vi "Chip.vi"() -> ()   [LabVIEW 2018]
uses:
  Controls/ClusterF.ctl
  Controls/OpcodeEnum.ctl
  <vilib>/picture/picture.llb/Draw 4-Bit Pixmap.vi
panel:
  out "Display":picture
  # "Keypad                   Keyboard\n+-+-+-+-+                +-+-+-+-+\n|1|2|3|C|                      |1|2|3|4|\n+-+-+-+-+                +-+-+-+-+\n|4|5|6|D|                      |Q|W|E|R|\n+-+-+-+-+     =>     +-+-+-+-+\n|7|8|9|E|                       |A|S|D|F|\n+-+-+-+-+                +-+-+-+-+\n|A|0|B|F|                      |Z|X|C|V|\n+-+-+-+-+                +-+-+-+-+"
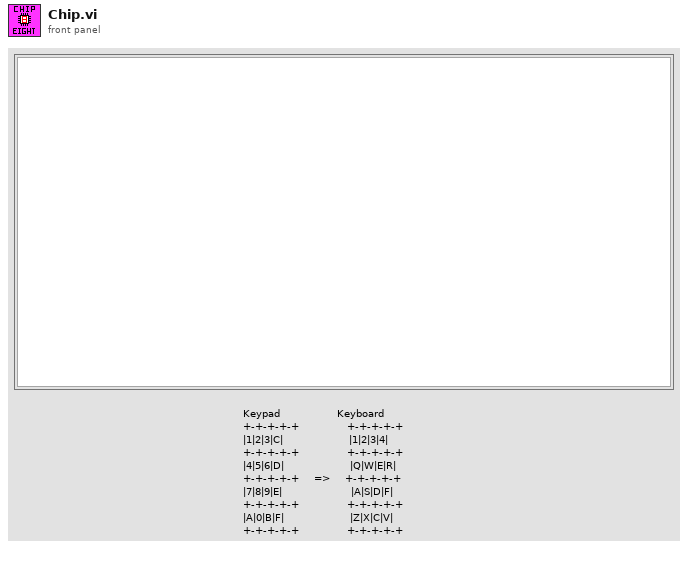
[diagram p1: front panel]
types:
  T1 = typedef "OpcodeEnum.ctl" = enum16{"Initialize", "Load ROM & Fontset", "Fetch Opcode", "Decode Opcode", "Update Display", "Execute Opcode", "Exit Program", "0NNN: Call", "00E0: Clear Display", "00EE: Return from subroutine", "1NNN: Jump to Addr NNN", "2NNN: Call subroutine at NNN", "3XNN: Skip if VX == NN", "4XNN: Skip if VX != NN", "5XY0: Skip if VX = VY", "6XNN: VX = NN", "7XNN: Add NN to VX", "8XY0: VX = VY", "8XY1: VX = VX or VY", "8XY2: VX = VX and VY", "8XY3: VX = VX xor VY", "8XY4: VX += VY", "8XY5: VY - VX", "8XY6: Sig bit of VX to VF, then shift right", "8XY7: Set VX = VY-VX", "8XYE: Sig bit of VX to VF, then shift VX left", "9XY0: Skip if VX != VY", "ANNN: Set I to Addr NNN", "BNNN: Jump to Addr NNN + V0", "CXNN: Set VX to result of rand", "DXYN: Draw Sprite at VX VY (OLD)", "DXYN: Draw Sprite at VX VY", "EX9E: Skip if key stored in VX is pressed", "EXA1: Skip if key stored in VX isn't pressed", "FX07: Set VX to value of DelayTimer", "FX0A: Keypress to VX blocking", "FX15: Set Delay Timer to VX", "FX18: Set SoundTimer to VX", "FX1E: Add VX to I", "FX29: Set Loc of Sprite for VX", "FX33: Store BCD of VX", "FX55: Store V0 to VX", "FX65: Fill V0 to VX", "Debug: Opcode Not Done Yet", "Undefined OpCode"}
  T2 = typedef "ClusterF.ctl" = cluster{"I":u16, "PC":u16, "Memory":u8[], "Keys":u8[], "V Registers":u8[], "Stack":u16[], "StackPointer":u16, "DelayTimer":u8, "SoundTimer":u8, "Display":u8[][], "Opcode":u16, "Display Coords":cluster{"X":u8, "Y":u8}, "GFX":u8[]}
  T3 = enum32{"invalid app kind", "Development System", "Run Time System", "Student Edition", "Embedded LabVIEW", "Evaluation", "Custom"}
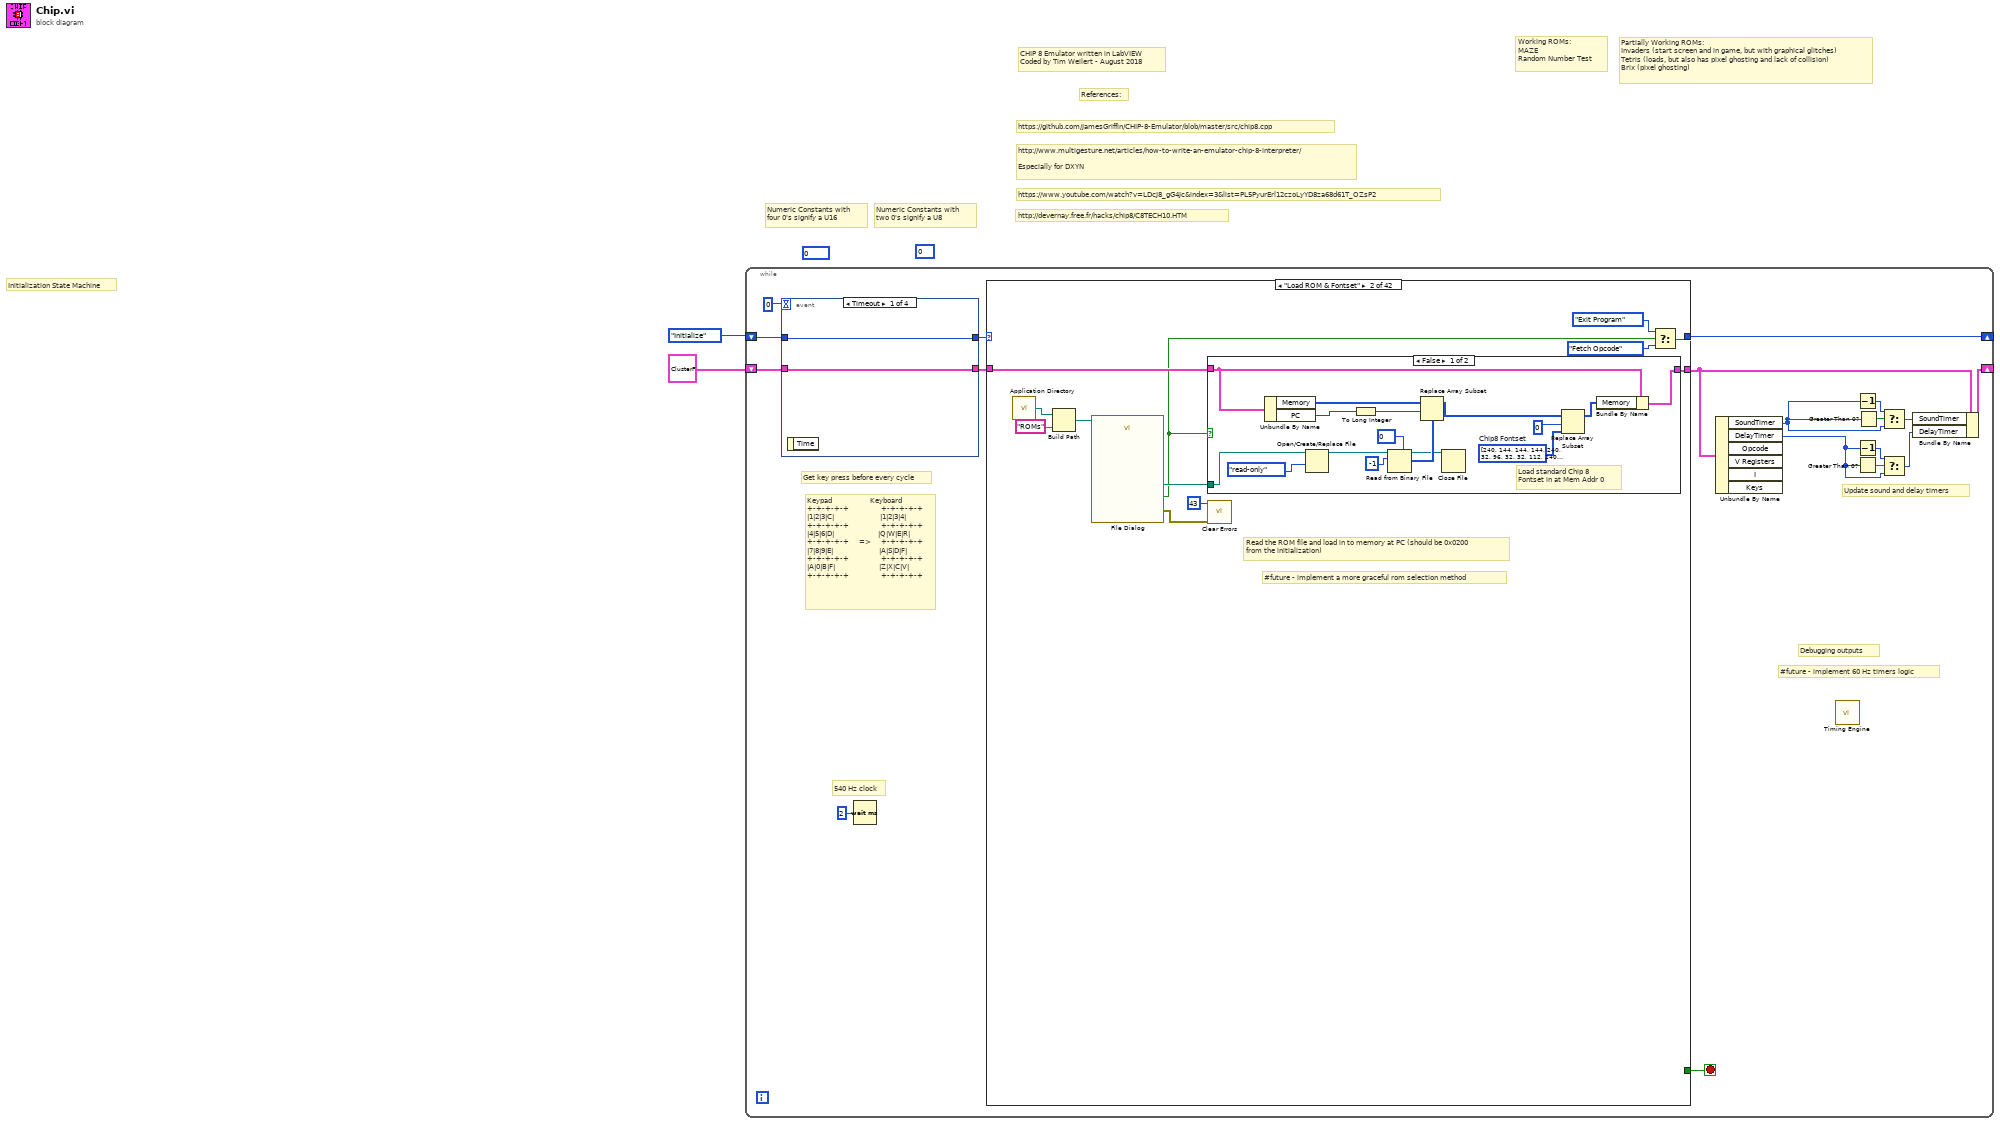
[diagram p0: block diagram]
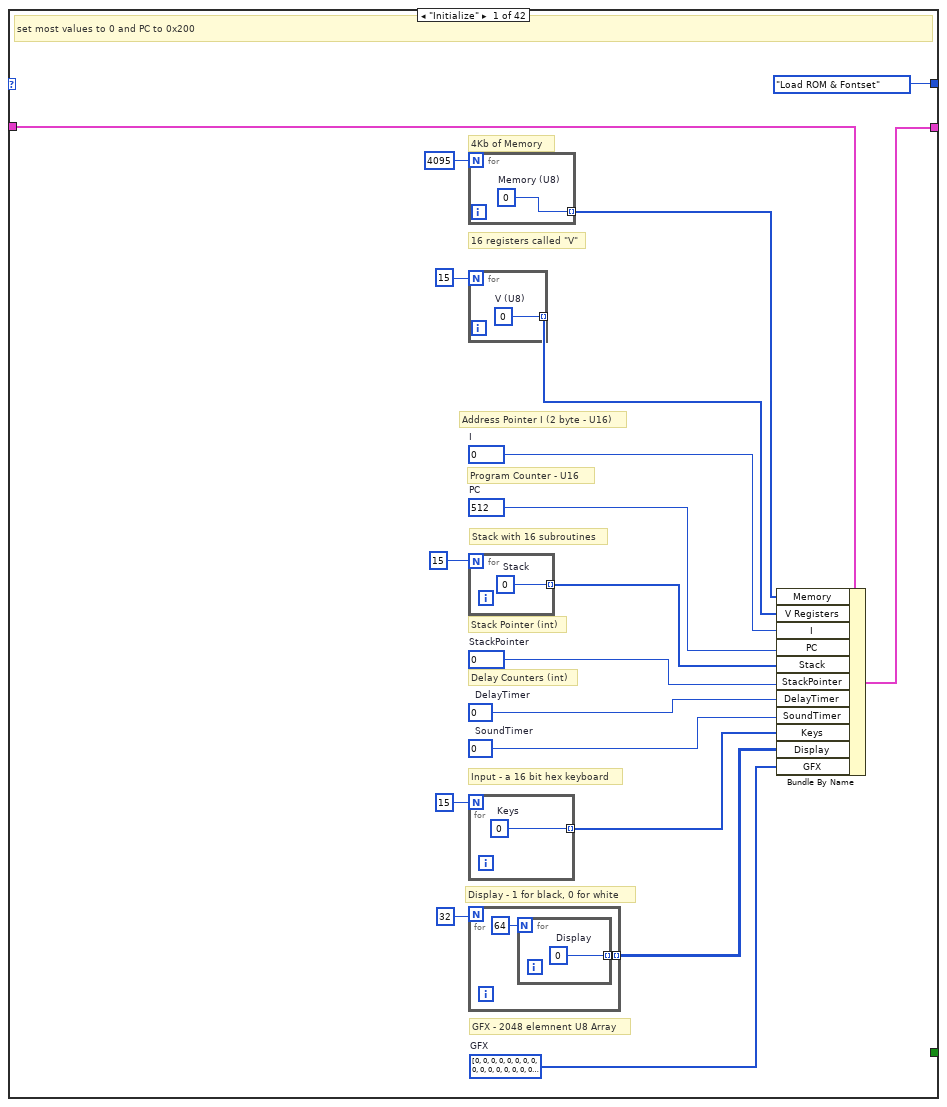
[diagram p2: hidden frame]
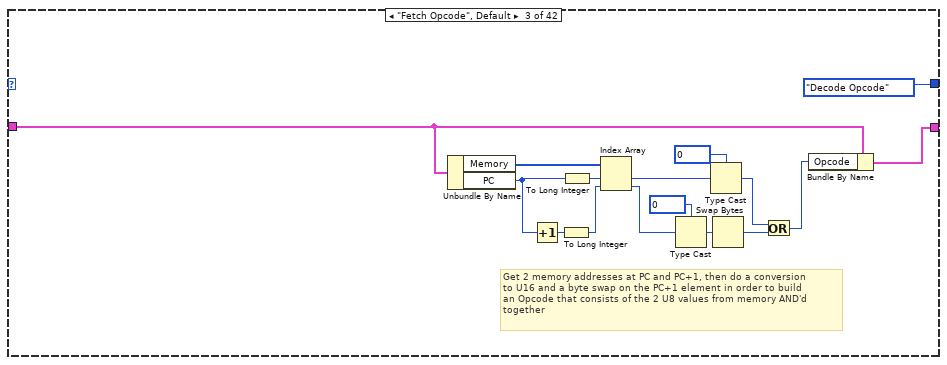
[diagram p4: hidden frame]
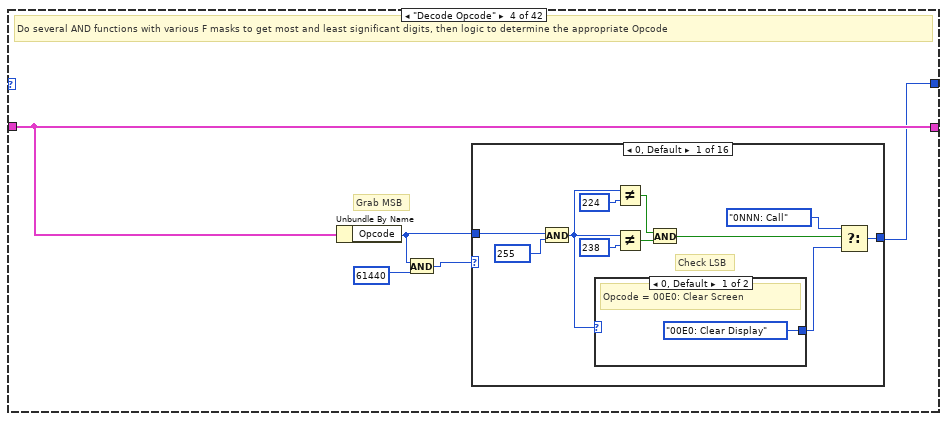
[diagram p5: hidden frame]
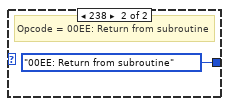
[diagram p6: hidden frame]
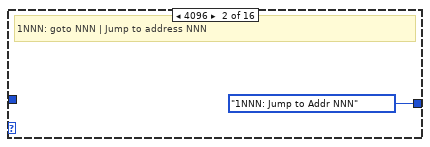
[diagram p7: hidden frame]
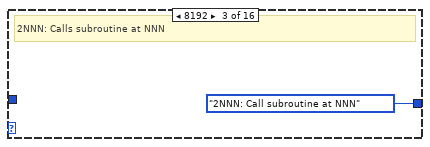
[diagram p8: hidden frame]
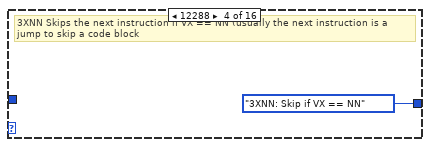
[diagram p9: hidden frame]
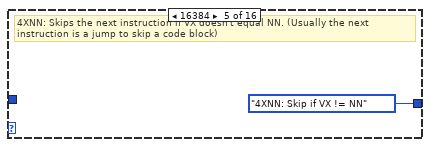
[diagram p10: hidden frame]
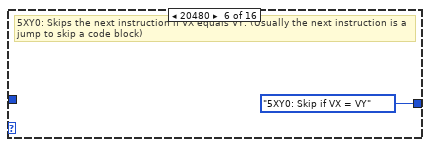
[diagram p11: hidden frame]
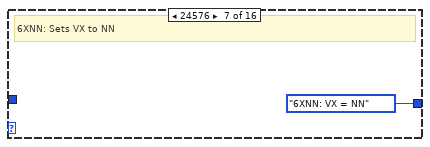
[diagram p12: hidden frame]
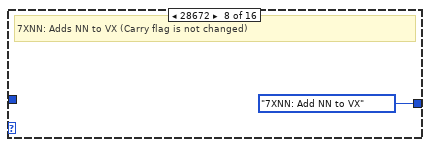
[diagram p13: hidden frame]
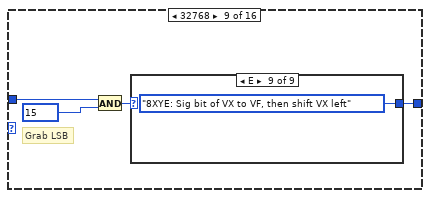
[diagram p14: hidden frame]
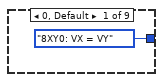
[diagram p15: hidden frame]
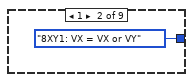
[diagram p16: hidden frame]
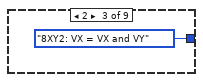
[diagram p17: hidden frame]
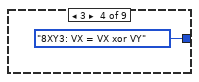
[diagram p18: hidden frame]
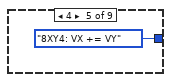
[diagram p19: hidden frame]
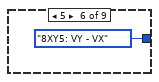
[diagram p20: hidden frame]
diagram:
  (unwired) u8 0
  (unwired) u16 0 ("y")
  # "Partially Working ROMs:\nInvaders (start screen and in game, but with graphical glitches)\nTetris (loads, but also has pixel ghosting and lack of collision)\nBrix (pixel ghosting)"
  # "Working ROMs:\nMAZE\nRandom Number Test"
  # "CHIP 8 Emulator written in LabVIEW\nCoded by Tim Weilert - August 2018"
  # "http://devernay.free.fr/hacks/chip8/C8TECH10.HTM"
  # "References:"
  # "Numeric Constants with \ntwo 0's signify a U8"
  # "Numeric Constants with \nfour 0's signify a U16"
  # "https://github.com/JamesGriffin/CHIP-8-Emulator/blob/master/src/chip8.cpp"
  # "http://www.multigesture.net/articles/how-to-write-an-emulator-chip-8-interpreter/\n\nEspecially for DXYN"
  # "https://www.youtube.com/watch?v=LDcJ8_gG4Jc&index=3&list=PL5PyurErl12czoLyYD8za68d61T_OZsP2"
  # "Initialization State Machine"
  n1 = while {
    shift-right: [w9] -> _
    shift-left: T2 {"I"=0, "PC"=0, "Memory"=array[4095 elements], "Keys"=[0, 0, 0, 0, 0, 0, 0, 0, 0, 0, 0, 0, 0, 0, 0], "V Registers"=[0, 0, 0, 0, 0, 0, 0, 0, 0, 0, 0, 0, 0, 0, 0], "Stack"=[0, 0, 0, 0, 0, 0, 0, 0, 0, 0, 0, 0, 0, 0, 0], "StackPointer"=0, "DelayTimer"=0, "SoundTimer"=0, "Display"=[[0, 0, 0, 0, 0, 0, 0, 0, 0, 0, 0, 0, 0, 0, 0, 0, 0, 0, 0, 0, 0, 0, 0, 0, 0, 0, 0, 0, 0, 0, 0, 0, 0, 0, 0, 0, 0, 0, 0, 0, 0, 0, 0, 0, 0, 0, 0, 0, 0, 0, 0, 0, 0, 0, 0, 0, 0, 0, 0, 0, 0, 0, 0, 0, 0], [0, 0, 0, 0, 0, 0, 0, 0, 0, 0, 0, 0, 0, 0, 0, 0, 0, 0, 0, 0, 0, 0, 0, 0, 0, 0, 0, 0, 0, 0, 0, 0, 0, 0, 0, 0, 0, 0, 0, 0, 0, 0, 0, 0, 0, 0, 0, 0, 0, 0, 0, 0, 0, 0, 0, 0, 0, 0, 0, 0, 0, 0, 0, 0, 0], [0, 0, 0, 0, 0, 0, 0, 0, 0, 0, 0, 0, 0, 0, 0, 0, 0, 0, 0, 0, 0, 0, 0, 0, 0, 0, 0, 0, 0, 0, 0, 0, 0, 0, 0, 0, 0, 0, 0, 0, 0, 0, 0, 0, 0, 0, 0, 0, 0, 0, 0, 0, 0, 0, 0, 0, 0, 0, 0, 0, 0, 0, 0, 0, 0], [0, 0, 0, 0, 0, 0, 0, 0, 0, 0, 0, 0, 0, 0, 0, 0, 0, 0, 0, 0, 0, 0, 0, 0, 0, 0, 0, 0, 0, 0, 0, 0, 0, 0, 0, 0, 0, 0, 0, 0, 0, 0, 0, 0, 0, 0, 0, 0, 0, 0, 0, 0, 0, 0, 0, 0, 0, 0, 0, 0, 0, 0, 0, 0, 0], [0, 0, 0, 0, 0, 0, 0, 0, 0, 0, 0, 0, 0, 0, 0, 0, 0, 0, 0, 0, 0, 0, 0, 0, 0, 0, 0, 0, 0, 0, 0, 0, 0, 0, 0, 0, 0, 0, 0, 0, 0, 0, 0, 0, 0, 0, 0, 0, 0, 0, 0, 0, 0, 0, 0, 0, 0, 0, 0, 0, 0, 0, 0, 0, 0], [0, 0, 0, 0, 0, 0, 0, 0, 0, 0, 0, 0, 0, 0, 0, 0, 0, 0, 0, 0, 0, 0, 0, 0, 0, 0, 0, 0, 0, 0, 0, 0, 0, 0, 0, 0, 0, 0, 0, 0, 0, 0, 0, 0, 0, 0, 0, 0, 0, 0, 0, 0, 0, 0, 0, 0, 0, 0, 0, 0, 0, 0, 0, 0, 0], [0, 0, 0, 0, 0, 0, 0, 0, 0, 0, 0, 0, 0, 0, 0, 0, 0, 0, 0, 0, 0, 0, 0, 0, 0, 0, 0, 0, 0, 0, 0, 0, 0, 0, 0, 0, 0, 0, 0, 0, 0, 0, 0, 0, 0, 0, 0, 0, 0, 0, 0, 0, 0, 0, 0, 0, 0, 0, 0, 0, 0, 0, 0, 0, 0], [0, 0, 0, 0, 0, 0, 0, 0, 0, 0, 0, 0, 0, 0, 0, 0, 0, 0, 0, 0, 0, 0, 0, 0, 0, 0, 0, 0, 0, 0, 0, 0, 0, 0, 0, 0, 0, 0, 0, 0, 0, 0, 0, 0, 0, 0, 0, 0, 0, 0, 0, 0, 0, 0, 0, 0, 0, 0, 0, 0, 0, 0, 0, 0, 0], [0, 0, 0, 0, 0, 0, 0, 0, 0, 0, 0, 0, 0, 0, 0, 0, 0, 0, 0, 0, 0, 0, 0, 0, 0, 0, 0, 0, 0, 0, 0, 0, 0, 0, 0, 0, 0, 0, 0, 0, 0, 0, 0, 0, 0, 0, 0, 0, 0, 0, 0, 0, 0, 0, 0, 0, 0, 0, 0, 0, 0, 0, 0, 0, 0], [0, 0, 0, 0, 0, 0, 0, 0, 0, 0, 0, 0, 0, 0, 0, 0, 0, 0, 0, 0, 0, 0, 0, 0, 0, 0, 0, 0, 0, 0, 0, 0, 0, 0, 0, 0, 0, 0, 0, 0, 0, 0, 0, 0, 0, 0, 0, 0, 0, 0, 0, 0, 0, 0, 0, 0, 0, 0, 0, 0, 0, 0, 0, 0, 0], [0, 0, 0, 0, 0, 0, 0, 0, 0, 0, 0, 0, 0, 0, 0, 0, 0, 0, 0, 0, 0, 0, 0, 0, 0, 0, 0, 0, 0, 0, 0, 0, 0, 0, 0, 0, 0, 0, 0, 0, 0, 0, 0, 0, 0, 0, 0, 0, 0, 0, 0, 0, 0, 0, 0, 0, 0, 0, 0, 0, 0, 0, 0, 0, 0], [0, 0, 0, 0, 0, 0, 0, 0, 0, 0, 0, 0, 0, 0, 0, 0, 0, 0, 0, 0, 0, 0, 0, 0, 0, 0, 0, 0, 0, 0, 0, 0, 0, 0, 0, 0, 0, 0, 0, 0, 0, 0, 0, 0, 0, 0, 0, 0, 0, 0, 0, 0, 0, 0, 0, 0, 0, 0, 0, 0, 0, 0, 0, 0, 0], [0, 0, 0, 0, 0, 0, 0, 0, 0, 0, 0, 0, 0, 0, 0, 0, 0, 0, 0, 0, 0, 0, 0, 0, 0, 0, 0, 0, 0, 0, 0, 0, 0, 0, 0, 0, 0, 0, 0, 0, 0, 0, 0, 0, 0, 0, 0, 0, 0, 0, 0, 0, 0, 0, 0, 0, 0, 0, 0, 0, 0, 0, 0, 0, 0], [0, 0, 0, 0, 0, 0, 0, 0, 0, 0, 0, 0, 0, 0, 0, 0, 0, 0, 0, 0, 0, 0, 0, 0, 0, 0, 0, 0, 0, 0, 0, 0, 0, 0, 0, 0, 0, 0, 0, 0, 0, 0, 0, 0, 0, 0, 0, 0, 0, 0, 0, 0, 0, 0, 0, 0, 0, 0, 0, 0, 0, 0, 0, 0, 0], [0, 0, 0, 0, 0, 0, 0, 0, 0, 0, 0, 0, 0, 0, 0, 0, 0, 0, 0, 0, 0, 0, 0, 0, 0, 0, 0, 0, 0, 0, 0, 0, 0, 0, 0, 0, 0, 0, 0, 0, 0, 0, 0, 0, 0, 0, 0, 0, 0, 0, 0, 0, 0, 0, 0, 0, 0, 0, 0, 0, 0, 0, 0, 0, 0], [0, 0, 0, 0, 0, 0, 0, 0, 0, 0, 0, 0, 0, 0, 0, 0, 0, 0, 0, 0, 0, 0, 0, 0, 0, 0, 0, 0, 0, 0, 0, 0, 0, 0, 0, 0, 0, 0, 0, 0, 0, 0, 0, 0, 0, 0, 0, 0, 0, 0, 0, 0, 0, 0, 0, 0, 0, 0, 0, 0, 0, 0, 0, 0, 0], [0, 0, 0, 0, 0, 0, 0, 0, 0, 0, 0, 0, 0, 0, 0, 0, 0, 0, 0, 0, 0, 0, 0, 0, 0, 0, 0, 0, 0, 0, 0, 0, 0, 0, 0, 0, 0, 0, 0, 0, 0, 0, 0, 0, 0, 0, 0, 0, 0, 0, 0, 0, 0, 0, 0, 0, 0, 0, 0, 0, 0, 0, 0, 0, 0], [0, 0, 0, 0, 0, 0, 0, 0, 0, 0, 0, 0, 0, 0, 0, 0, 0, 0, 0, 0, 0, 0, 0, 0, 0, 0, 0, 0, 0, 0, 0, 0, 0, 0, 0, 0, 0, 0, 0, 0, 0, 0, 0, 0, 0, 0, 0, 0, 0, 0, 0, 0, 0, 0, 0, 0, 0, 0, 0, 0, 0, 0, 0, 0, 0], [0, 0, 0, 0, 0, 0, 0, 0, 0, 0, 0, 0, 0, 0, 0, 0, 0, 0, 0, 0, 0, 0, 0, 0, 0, 0, 0, 0, 0, 0, 0, 0, 0, 0, 0, 0, 0, 0, 0, 0, 0, 0, 0, 0, 0, 0, 0, 0, 0, 0, 0, 0, 0, 0, 0, 0, 0, 0, 0, 0, 0, 0, 0, 0, 0], [0, 0, 0, 0, 0, 0, 0, 0, 0, 0, 0, 0, 0, 0, 0, 0, 0, 0, 0, 0, 0, 0, 0, 0, 0, 0, 0, 0, 0, 0, 0, 0, 0, 0, 0, 0, 0, 0, 0, 0, 0, 0, 0, 0, 0, 0, 0, 0, 0, 0, 0, 0, 0, 0, 0, 0, 0, 0, 0, 0, 0, 0, 0, 0, 0], [0, 0, 0, 0, 0, 0, 0, 0, 0, 0, 0, 0, 0, 0, 0, 0, 0, 0, 0, 0, 0, 0, 0, 0, 0, 0, 0, 0, 0, 0, 0, 0, 0, 0, 0, 0, 0, 0, 0, 0, 0, 0, 0, 0, 0, 0, 0, 0, 0, 0, 0, 0, 0, 0, 0, 0, 0, 0, 0, 0, 0, 0, 0, 0, 0], [0, 0, 0, 0, 0, 0, 0, 0, 0, 0, 0, 0, 0, 0, 0, 0, 0, 0, 0, 0, 0, 0, 0, 0, 0, 0, 0, 0, 0, 0, 0, 0, 0, 0, 0, 0, 0, 0, 0, 0, 0, 0, 0, 0, 0, 0, 0, 0, 0, 0, 0, 0, 0, 0, 0, 0, 0, 0, 0, 0, 0, 0, 0, 0, 0], [0, 0, 0, 0, 0, 0, 0, 0, 0, 0, 0, 0, 0, 0, 0, 0, 0, 0, 0, 0, 0, 0, 0, 0, 0, 0, 0, 0, 0, 0, 0, 0, 0, 0, 0, 0, 0, 0, 0, 0, 0, 0, 0, 0, 0, 0, 0, 0, 0, 0, 0, 0, 0, 0, 0, 0, 0, 0, 0, 0, 0, 0, 0, 0, 0], [0, 0, 0, 0, 0, 0, 0, 0, 0, 0, 0, 0, 0, 0, 0, 0, 0, 0, 0, 0, 0, 0, 0, 0, 0, 0, 0, 0, 0, 0, 0, 0, 0, 0, 0, 0, 0, 0, 0, 0, 0, 0, 0, 0, 0, 0, 0, 0, 0, 0, 0, 0, 0, 0, 0, 0, 0, 0, 0, 0, 0, 0, 0, 0, 0], [0, 0, 0, 0, 0, 0, 0, 0, 0, 0, 0, 0, 0, 0, 0, 0, 0, 0, 0, 0, 0, 0, 0, 0, 0, 0, 0, 0, 0, 0, 0, 0, 0, 0, 0, 0, 0, 0, 0, 0, 0, 0, 0, 0, 0, 0, 0, 0, 0, 0, 0, 0, 0, 0, 0, 0, 0, 0, 0, 0, 0, 0, 0, 0, 0], [0, 0, 0, 0, 0, 0, 0, 0, 0, 0, 0, 0, 0, 0, 0, 0, 0, 0, 0, 0, 0, 0, 0, 0, 0, 0, 0, 0, 0, 0, 0, 0, 0, 0, 0, 0, 0, 0, 0, 0, 0, 0, 0, 0, 0, 0, 0, 0, 0, 0, 0, 0, 0, 0, 0, 0, 0, 0, 0, 0, 0, 0, 0, 0, 0], [0, 0, 0, 0, 0, 0, 0, 0, 0, 0, 0, 0, 0, 0, 0, 0, 0, 0, 0, 0, 0, 0, 0, 0, 0, 0, 0, 0, 0, 0, 0, 0, 0, 0, 0, 0, 0, 0, 0, 0, 0, 0, 0, 0, 0, 0, 0, 0, 0, 0, 0, 0, 0, 0, 0, 0, 0, 0, 0, 0, 0, 0, 0, 0, 0], [0, 0, 0, 0, 0, 0, 0, 0, 0, 0, 0, 0, 0, 0, 0, 0, 0, 0, 0, 0, 0, 0, 0, 0, 0, 0, 0, 0, 0, 0, 0, 0, 0, 0, 0, 0, 0, 0, 0, 0, 0, 0, 0, 0, 0, 0, 0, 0, 0, 0, 0, 0, 0, 0, 0, 0, 0, 0, 0, 0, 0, 0, 0, 0, 0], [0, 0, 0, 0, 0, 0, 0, 0, 0, 0, 0, 0, 0, 0, 0, 0, 0, 0, 0, 0, 0, 0, 0, 0, 0, 0, 0, 0, 0, 0, 0, 0, 0, 0, 0, 0, 0, 0, 0, 0, 0, 0, 0, 0, 0, 0, 0, 0, 0, 0, 0, 0, 0, 0, 0, 0, 0, 0, 0, 0, 0, 0, 0, 0, 0], [0, 0, 0, 0, 0, 0, 0, 0, 0, 0, 0, 0, 0, 0, 0, 0, 0, 0, 0, 0, 0, 0, 0, 0, 0, 0, 0, 0, 0, 0, 0, 0, 0, 0, 0, 0, 0, 0, 0, 0, 0, 0, 0, 0, 0, 0, 0, 0, 0, 0, 0, 0, 0, 0, 0, 0, 0, 0, 0, 0, 0, 0, 0, 0, 0], [0, 0, 0, 0, 0, 0, 0, 0, 0, 0, 0, 0, 0, 0, 0, 0, 0, 0, 0, 0, 0, 0, 0, 0, 0, 0, 0, 0, 0, 0, 0, 0, 0, 0, 0, 0, 0, 0, 0, 0, 0, 0, 0, 0, 0, 0, 0, 0, 0, 0, 0, 0, 0, 0, 0, 0, 0, 0, 0, 0, 0, 0, 0, 0, 0], [0, 0, 0, 0, 0, 0, 0, 0, 0, 0, 0, 0, 0, 0, 0, 0, 0, 0, 0, 0, 0, 0, 0, 0, 0, 0, 0, 0, 0, 0, 0, 0, 0, 0, 0, 0, 0, 0, 0, 0, 0, 0, 0, 0, 0, 0, 0, 0, 0, 0, 0, 0, 0, 0, 0, 0, 0, 0, 0, 0, 0, 0, 0, 0, 0], [0, 0, 0, 0, 0, 0, 0, 0, 0, 0, 0, 0, 0, 0, 0, 0, 0, 0, 0, 0, 0, 0, 0, 0, 0, 0, 0, 0, 0, 0, 0, 0, 0, 0, 0, 0, 0, 0, 0, 0, 0, 0, 0, 0, 0, 0, 0, 0, 0, 0, 0, 0, 0, 0, 0, 0, 0, 0, 0, 0, 0, 0, 0, 0, 0]], "Opcode"=0, "Display Coords"={"X"=0, "Y"=0}, "GFX"=[]} ("Variables and Memory") -> [w18]
    shift-right: [w5] -> _
    shift-left: OpcodeEnum."Initialize" -> [w4]
    stop <- w20 stop-if-true
    # "#future - implement 60 Hz timers logic"
    # "Debugging outputs"
    # "Update sound and delay timers"
    # "540 Hz clock"
    # "Get key press before every cycle"
    # "Keypad                   Keyboard\n+-+-+-+-+                +-+-+-+-+\n|1|2|3|C|                       |1|2|3|4|\n+-+-+-+-+                +-+-+-+-+\n|4|5|6|D|                      |Q|W|E|R|\n+-+-+-+-+     =>     +-+-+-+-+\n|7|8|9|E|                       |A|S|D|F|\n+-+-+-+-+                +-+-+-+-+\n|A|0|B|F|                      |Z|X|C|V|\n+-+-+-+-+                +-+-+-+-+"
    n2 = event shown="[0] Timeout" {
      selector: _ -> [_ _ _ _]
      dyn-events: _ -> [_ _ _ _]
      timeout: 0 -> [_ _ _ _]
      tunnel: w18 -> [w788 w789 w795 w799]
      tunnel: [w788 w789 w793 w800] -> w17
      tunnel: w4 -> [w787 _ w792 w796]
      tunnel: [w787 OpcodeEnum."Exit Program" w792 w796] -> w3
      event Timeout {
        n3 = event-data() -> ()  [unwired: 1 in, 1 out]
      }
      event Panel Close? {
        n4 = event-data() -> ()  [unwired: 1 in, 1 out]
        n5 = event-data("Discard?"=TRUE) -> ()  [unwired: 1 in, 1 out]
      }
      event Key Up {
        n6 = event-data() -> ()  [unwired: 1 in, 1 out]
        n7 = Bundle By Name(cluster=w795, "Keys"=u8[] [0, 0, 0, 0, 0, 0, 0, 0, 0, 0, 0, 0, 0, 0, 0, 0]) -> (w793:T2)
      }
      event Key Down {
        n8 = event-data() -> ("Char"=w798:i16)  [unwired: 1 in]
        n9 = case shown="78" w798 {
          tunnel: [u8[] [0, 0, 0, 0, 0, 0, 0, 0, 0, 0, 0, 0, 0, 0, 0, 0] ("Keys 2") u8[] [0, 1, 0, 0, 0, 0, 0, 0, 0, 0, 0, 0, 0, 0, 0, 0] ("Keys 2") u8[] [0, 0, 1, 0, 0, 0, 0, 0, 0, 0, 0, 0, 0, 0, 0, 0] ("Keys 2") u8[] [0, 0, 0, 1, 0, 0, 0, 0, 0, 0, 0, 0, 0, 0, 0, 0] ("Keys 2") u8[] [0, 0, 0, 0, 0, 0, 0, 0, 0, 0, 0, 0, 1, 0, 0, 0] ("Keys 2") u8[] [0, 0, 0, 0, 1, 0, 0, 0, 0, 0, 0, 0, 0, 0, 0, 0] ("Keys 2") u8[] [0, 0, 0, 0, 0, 1, 0, 0, 0, 0, 0, 0, 0, 0, 0, 0] ("Keys 2") u8[] [0, 0, 0, 0, 0, 0, 1, 0, 0, 0, 0, 0, 0, 0, 0, 0] ("Keys 2") u8[] [0, 0, 0, 0, 0, 0, 0, 0, 0, 0, 0, 0, 0, 1, 0, 0] ("Keys 2") u8[] [0, 0, 0, 0, 0, 0, 0, 1, 0, 0, 0, 0, 0, 0, 0, 0] ("Keys 2") u8[] [0, 0, 0, 0, 0, 0, 0, 0, 1, 0, 0, 0, 0, 0, 0, 0] ("Keys 2") u8[] [0, 0, 0, 0, 0, 0, 0, 0, 0, 1, 0, 0, 0, 0, 0, 0] ("Keys 2") u8[] [0, 0, 0, 0, 0, 0, 0, 0, 0, 0, 0, 0, 0, 0, 1, 0] ("Keys 2") u8[] [0, 0, 0, 0, 0, 0, 0, 0, 0, 0, 1, 0, 0, 0, 0, 0] ("Keys 2") u8[] [1, 0, 0, 0, 0, 0, 0, 0, 0, 0, 0, 0, 0, 0, 0, 0] ("Keys 2") u8[] [0, 0, 0, 0, 0, 0, 0, 0, 0, 0, 0, 1, 0, 0, 0, 0] ("Keys 2") u8[] [0, 0, 0, 0, 0, 0, 0, 0, 0, 0, 0, 0, 0, 0, 0, 1] ("Keys 2")] -> w797
          frame 0, Default {
          }
          frame 49 {
            # "1 = 1"
          }
          frame 50 {
            # "2 = 2"
          }
          frame 51 {
            # "3 = 3"
          }
          frame 52 {
            # "4 =C"
          }
          frame 113 {
            # "Q = 4"
          }
          frame 119 {
            # "W = 5"
          }
          frame 101 {
            # "E = 6"
          }
          frame 114 {
            # "R = D"
          }
          frame 97 {
            # "A = 7"
          }
          frame 115 {
            # "S = 8"
          }
          frame 100 {
            # "D = 9"
          }
          frame 102 {
            # "F = E"
          }
          frame 122 {
            # "Z = A"
          }
          frame 120 {
            # "X = 0"
          }
          frame 99 {
            # "C = B"
          }
          frame 118 {
            # "V = F"
          }
        }
        n10 = Bundle By Name(cluster=w799, "Keys"=w797) -> (w800:T2)
      }
    }
    n11 = Wait (ms)(milliseconds to wait=u32 2) -> ()  [unwired: 1 out]
    n12 = case shown="\"Load ROM & Fontset\"" w3 {
      tunnel: w17 -> [w22 w58 w89 w96 w159 w162 w167 w177 w189 w198 w205 w226 w235 w259 w275 w285 w308 w328 w338 w354 w384 w402 w423 w453 w474 w495 w507 w511 w530 w546 w557 w585 w599 w602 w652 w657 w685 w702 w735 w754 w771 w783]
      tunnel: [w23 w57 w88 w96 w159 w162 w168 w178 w190 w197 w206 w227 w233 w258 w276 w286 w309 w327 w337 w355 w385 w401 w422 w454 w473 w494 w508 w512 w531 w548 w558 w584 w600 w608 w653 w658 w686 w703 w736 w755 w770 w783] -> w10
      tunnel: [OpcodeEnum."Load ROM & Fontset" w50 OpcodeEnum."Decode Opcode" w93 OpcodeEnum."Fetch Opcode" OpcodeEnum."Exit Program" OpcodeEnum."Fetch Opcode" OpcodeEnum."Update Display" OpcodeEnum."Fetch Opcode" OpcodeEnum."Fetch Opcode" OpcodeEnum."Fetch Opcode" OpcodeEnum."Fetch Opcode" OpcodeEnum."Fetch Opcode" OpcodeEnum."Fetch Opcode" OpcodeEnum."Fetch Opcode" OpcodeEnum."Fetch Opcode" OpcodeEnum."Fetch Opcode" OpcodeEnum."Fetch Opcode" OpcodeEnum."Fetch Opcode" OpcodeEnum."Fetch Opcode" OpcodeEnum."Fetch Opcode" OpcodeEnum."Fetch Opcode" OpcodeEnum."Fetch Opcode" OpcodeEnum."Fetch Opcode" OpcodeEnum."Fetch Opcode" OpcodeEnum."Fetch Opcode" OpcodeEnum."Fetch Opcode" OpcodeEnum."Fetch Opcode" OpcodeEnum."Fetch Opcode" OpcodeEnum."Update Display" OpcodeEnum."Fetch Opcode" OpcodeEnum."Fetch Opcode" OpcodeEnum."Fetch Opcode" OpcodeEnum."Fetch Opcode" OpcodeEnum."Fetch Opcode" OpcodeEnum."Fetch Opcode" OpcodeEnum."Fetch Opcode" OpcodeEnum."Fetch Opcode" OpcodeEnum."Fetch Opcode" OpcodeEnum."Fetch Opcode" OpcodeEnum."Fetch Opcode" OpcodeEnum."Debug: Opcode Not Done Yet"] -> w5
      tunnel: [_ _ _ _ _ TRUE _ _ _ _ _ _ _ _ _ _ _ _ _ _ _ _ _ _ _ _ _ _ _ FALSE _ _ _ _ _ _ _ _ _ _ _ TRUE] -> w20
      frame "Initialize" {
        w24 = u8[] [0, 0, 0, 0, 0, 0, 0, 0, 0, 0, 0, 0, 0, 0, 0, 0, 0, 0, 0, 0, 0, 0, 0, 0, 0, 0, 0, 0, 0, 0, 0, 0, 0, 0, 0, 0, 0, 0, 0, 0, 0, 0, 0, 0, 0, 0, 0, 0, 0, 0, 0, 0, 0, 0, 0, 0, 0, 0, 0, 0, 0, 0, 0, 0, 0, 0, 0, 0, 0, 0, 0, 0, 0, 0, 0, 0, 0, 0, 0, 0, 0, 0, 0, 0, 0, 0, 0, 0, 0, 0, 0, 0, 0, 0, 0, 0, 0, 0, 0, 0, 0, 0, 0, 0, 0, 0, 0, 0, 0, 0, 0, 0, 0, 0, 0, 0, 0, 0, 0, 0, 0, 0, 0, 0, 0, 0, 0, 0, 0, 0, 0, 0, 0, 0, 0, 0, 0, 0, 0, 0, 0, 0, 0, 0, 0, 0, 0, 0, 0, 0, 0, 0, 0, 0, 0, 0, 0, 0, 0, 0, 0, 0, 0, 0, 0, 0, 0, 0, 0, 0, 0, 0, 0, 0, 0, 0, 0, 0, 0, 0, 0, 0, 0, 0, 0, 0, 0, 0, 0, 0, 0, 0, 0, 0, 0, 0, 0, 0, 0, 0, 0, 0, 0, 0, 0, 0, 0, 0, 0, 0, 0, 0, 0, 0, 0, 0, 0, 0, 0, 0, 0, 0, 0, 0, 0, 0, 0, 0, 0, 0, 0, 0, 0, 0, 0, 0, 0, 0, 0, 0, 0, 0, 0, 0, 0, 0, 0, 0, 0, 0, 0, 0, 0, 0, 0, 0, 0, 0, 0, 0, 0, 0, 0, 0, 0, 0, 0, 0, 0, 0, 0, 0, 0, 0, 0, 0, 0, 0, 0, 0, 0, 0, 0, 0, 0, 0, 0, 0, 0, 0, 0, 0, 0, 0, 0, 0, 0, 0, 0, 0, 0, 0, 0, 0, 0, 0, 0, 0, 0, 0, 0, 0, 0, 0, 0, 0, 0, 0, 0, 0, 0, 0, 0, 0, 0, 0, 0, 0, 0, 0, 0, 0, 0, 0, 0, 0, 0, 0, 0, 0, 0, 0, 0, 0, 0, 0, 0, 0, 0, 0, 0, 0, 0, 0, 0, 0, 0, 0, 0, 0, 0, 0, 0, 0, 0, 0, 0, 0, 0, 0, 0, 0, 0, 0, 0, 0, 0, 0, 0, 0, 0, 0, 0, 0, 0, 0, 0, 0, 0, 0, 0, 0, 0, 0, 0, 0, 0, 0, 0, 0, 0, 0, 0, 0, 0, 0, 0, 0, 0, 0, 0, 0, 0, 0, 0, 0, 0, 0, 0, 0, 0, 0, 0, 0, 0, 0, 0, 0, 0, 0, 0, 0, 0, 0, 0, 0, 0, 0, 0, 0, 0, 0, 0, 0, 0, 0, 0, 0, 0, 0, 0, 0, 0, 0, 0, 0, 0, 0, 0, 0, 0, 0, 0, 0, 0, 0, 0, 0, 0, 0, 0, 0, 0, 0, 0, 0, 0, 0, 0, 0, 0, 0, 0, 0, 0, 0, 0, 0, 0, 0, 0, 0, 0, 0, 0, 0, 0, 0, 0, 0, 0, 0, 0, 0, 0, 0, 0, 0, 0, 0, 0, 0, 0, 0, 0, 0, 0, 0, 0, 0, 0, 0, 0, 0, 0, 0, 0, 0, 0, 0, 0, 0, 0, 0, 0, 0, 0, 0, 0, 0, 0, 0, 0, 0, 0, 0, 0, 0, 0, 0, 0, 0, 0, 0, 0, 0, 0, 0, 0, 0, 0, 0, 0, 0, 0, 0, 0, 0, 0, 0, 0, 0, 0, 0, 0, 0, 0, 0, 0, 0, 0, 0, 0, 0, 0, 0, 0, 0, 0, 0, 0, 0, 0, 0, 0, 0, 0, 0, 0, 0, 0, 0, 0, 0, 0, 0, 0, 0, 0, 0, 0, 0, 0, 0, 0, 0, 0, 0, 0, 0, 0, 0, 0, 0, 0, 0, 0, 0, 0, 0, 0, 0, 0, 0, 0, 0, 0, 0, 0, 0, 0, 0, 0, 0, 0, 0, 0, 0, 0, 0, 0, 0, 0, 0, 0, 0, 0, 0, 0, 0, 0, 0, 0, 0, 0, 0, 0, 0, 0, 0, 0, 0, 0, 0, 0, 0, 0, 0, 0, 0, 0, 0, 0, 0, 0, 0, 0, 0, 0, 0, 0, 0, 0, 0, 0, 0, 0, 0, 0, 0, 0, 0, 0, 0, 0, 0, 0, 0, 0, 0, 0, 0, 0, 0, 0, 0, 0, 0, 0, 0, 0, 0, 0, 0, 0, 0, 0, 0, 0, 0, 0, 0, 0, 0, 0, 0, 0, 0, 0, 0, 0, 0, 0, 0, 0, 0, 0, 0, 0, 0, 0, 0, 0, 0, 0, 0, 0, 0, 0, 0, 0, 0, 0, 0, 0, 0, 0, 0, 0, 0, 0, 0, 0, 0, 0, 0, 0, 0, 0, 0, 0, 0, 0, 0, 0, 0, 0, 0, 0, 0, 0, 0, 0, 0, 0, 0, 0, 0, 0, 0, 0, 0, 0, 0, 0, 0, 0, 0, 0, 0, 0, 0, 0, 0, 0, 0, 0, 0, 0, 0, 0, 0, 0, 0, 0, 0, 0, 0, 0, 0, 0, 0, 0, 0, 0, 0, 0, 0, 0, 0, 0, 0, 0, 0, 0, 0, 0, 0, 0, 0, 0, 0, 0, 0, 0, 0, 0, 0, 0, 0, 0, 0, 0, 0, 0, 0, 0, 0, 0, 0, 0, 0, 0, 0, 0, 0, 0, 0, 0, 0, 0, 0, 0, 0, 0, 0, 0, 0, 0, 0, 0, 0, 0, 0, 0, 0, 0, 0, 0, 0, 0, 0, 0, 0, 0, 0, 0, 0, 0, 0, 0, 0, 0, 0, 0, 0, 0, 0, 0, 0, 0, 0, 0, 0, 0, 0, 0, 0, 0, 0, 0, 0, 0, 0, 0, 0, 0, 0, 0, 0, 0, 0, 0, 0, 0, 0, 0, 0, 0, 0, 0, 0, 0, 0, 0, 0, 0, 0, 0, 0, 0, 0, 0, 0, 0, 0, 0, 0, 0, 0, 0, 0, 0, 0, 0, 0, 0, 0, 0, 0, 0, 0, 0, 0, 0, 0, 0, 0, 0, 0, 0, 0, 0, 0, 0, 0, 0, 0, 0, 0, 0, 0, 0, 0, 0, 0, 0, 0, 0, 0, 0, 0, 0, 0, 0, 0, 0, 0, 0, 0, 0, 0, 0, 0, 0, 0, 0, 0, 0, 0, 0, 0, 0, 0, 0, 0, 0, 0, 0, 0, 0, 0, 0, 0, 0, 0, 0, 0, 0, 0, 0, 0, 0, 0, 0, 0, 0, 0, 0, 0, 0, 0, 0, 0, 0, 0, 0, 0, 0, 0, 0, 0, 0, 0, 0, 0, 0, 0, 0, 0, 0, 0, 0, 0, 0, 0, 0, 0, 0, 0, 0, 0, 0, 0, 0, 0, 0, 0, 0, 0, 0, 0, 0, 0, 0, 0, 0, 0, 0, 0, 0, 0, 0, 0, 0, 0, 0, 0, 0, 0, 0, 0, 0, 0, 0, 0, 0, 0, 0, 0, 0, 0, 0, 0, 0, 0, 0, 0, 0, 0, 0, 0, 0, 0, 0, 0, 0, 0, 0, 0, 0, 0, 0, 0, 0, 0, 0, 0, 0, 0, 0, 0, 0, 0, 0, 0, 0, 0, 0, 0, 0, 0, 0, 0, 0, 0, 0, 0, 0, 0, 0, 0, 0, 0, 0, 0, 0, 0, 0, 0, 0, 0, 0, 0, 0, 0, 0, 0, 0, 0, 0, 0, 0, 0, 0, 0, 0, 0, 0, 0, 0, 0, 0, 0, 0, 0, 0, 0, 0, 0, 0, 0, 0, 0, 0, 0, 0, 0, 0, 0, 0, 0, 0, 0, 0, 0, 0, 0, 0, 0, 0, 0, 0, 0, 0, 0, 0, 0, 0, 0, 0, 0, 0, 0, 0, 0, 0, 0, 0, 0, 0, 0, 0, 0, 0, 0, 0, 0, 0, 0, 0, 0, 0, 0, 0, 0, 0, 0, 0, 0, 0, 0, 0, 0, 0, 0, 0, 0, 0, 0, 0, 0, 0, 0, 0, 0, 0, 0, 0, 0, 0, 0, 0, 0, 0, 0, 0, 0, 0, 0, 0, 0, 0, 0, 0, 0, 0, 0, 0, 0, 0, 0, 0, 0, 0, 0, 0, 0, 0, 0, 0, 0, 0, 0, 0, 0, 0, 0, 0, 0, 0, 0, 0, 0, 0, 0, 0, 0, 0, 0, 0, 0, 0, 0, 0, 0, 0, 0, 0, 0, 0, 0, 0, 0, 0, 0, 0, 0, 0, 0, 0, 0, 0, 0, 0, 0, 0, 0, 0, 0, 0, 0, 0, 0, 0, 0, 0, 0, 0, 0, 0, 0, 0, 0, 0, 0, 0, 0, 0, 0, 0, 0, 0, 0, 0, 0, 0, 0, 0, 0, 0, 0, 0, 0, 0, 0, 0, 0, 0, 0, 0, 0, 0, 0, 0, 0, 0, 0, 0, 0, 0, 0, 0, 0, 0, 0, 0, 0, 0, 0, 0, 0, 0, 0, 0, 0, 0, 0, 0, 0, 0, 0, 0, 0, 0, 0, 0, 0, 0, 0, 0, 0, 0, 0, 0, 0, 0, 0, 0, 0, 0, 0, 0, 0, 0, 0, 0, 0, 0, 0, 0, 0, 0, 0, 0, 0, 0, 0, 0, 0, 0, 0, 0, 0, 0, 0, 0, 0, 0, 0, 0, 0, 0, 0, 0, 0, 0, 0, 0, 0, 0, 0, 0, 0, 0, 0, 0, 0, 0, 0, 0, 0, 0, 0, 0, 0, 0, 0, 0, 0, 0, 0, 0, 0, 0, 0, 0, 0, 0, 0, 0, 0, 0, 0, 0, 0, 0, 0, 0, 0, 0, 0, 0, 0, 0, 0, 0, 0, 0, 0, 0, 0, 0, 0, 0, 0, 0, 0, 0, 0, 0, 0, 0, 0, 0, 0, 0, 0, 0, 0, 0, 0, 0, 0, 0, 0, 0, 0, 0, 0, 0, 0, 0, 0, 0, 0, 0, 0, 0, 0, 0, 0, 0, 0, 0, 0, 0, 0, 0, 0, 0, 0, 0, 0, 0, 0, 0, 0, 0, 0, 0, 0, 0, 0, 0, 0, 0, 0, 0, 0, 0, 0, 0, 0, 0, 0, 0, 0, 0, 0, 0, 0, 0, 0, 0, 0, 0, 0, 0, 0, 0, 0, 0, 0, 0, 0, 0, 0, 0, 0, 0, 0, 0, 0, 0, 0, 0, 0, 0, 0, 0, 0, 0, 0, 0, 0, 0, 0, 0, 0, 0, 0, 0, 0, 0, 0, 0, 0, 0, 0, 0, 0, 0, 0, 0, 0, 0, 0, 0, 0, 0, 0, 0, 0, 0, 0, 0, 0, 0, 0, 0, 0, 0, 0, 0, 0, 0, 0, 0, 0, 0, 0, 0, 0, 0, 0, 0, 0, 0, 0, 0, 0, 0, 0, 0, 0, 0, 0, 0, 0, 0, 0, 0, 0, 0, 0, 0, 0, 0, 0, 0, 0, 0, 0, 0, 0, 0, 0, 0, 0, 0, 0, 0, 0, 0, 0, 0, 0, 0, 0, 0, 0, 0, 0, 0, 0, 0, 0, 0, 0, 0, 0, 0, 0, 0, 0, 0, 0, 0, 0, 0, 0, 0, 0, 0, 0, 0, 0, 0, 0, 0, 0, 0, 0, 0, 0, 0, 0, 0, 0, 0, 0, 0, 0, 0, 0, 0, 0, 0, 0, 0, 0, 0, 0, 0, 0, 0, 0, 0, 0, 0, 0, 0, 0, 0, 0, 0, 0, 0, 0, 0, 0, 0, 0, 0, 0, 0, 0, 0, 0, 0, 0, 0, 0, 0, 0, 0, 0, 0, 0, 0, 0, 0, 0, 0, 0, 0, 0, 0, 0, 0, 0, 0, 0, 0, 0, 0, 0, 0, 0, 0, 0, 0, 0, 0, 0, 0, 0, 0, 0, 0, 0, 0, 0, 0, 0, 0, 0, 0, 0, 0, 0, 0, 0, 0, 0, 0, 0, 0, 0, 0, 0, 0, 0, 0, 0, 0, 0, 0, 0, 0, 0, 0, 0, 0, 0, 0, 0, 0, 0, 0, 0, 0, 0, 0, 0, 0, 0, 0, 0, 0, 0, 0, 0, 0, 0, 0, 0, 0, 0, 0, 0, 0, 0, 0, 0, 0, 0, 0, 0, 0, 0, 0, 0, 0, 0, 0, 0, 0, 0, 0, 0, 0, 0, 0, 0, 0, 0, 0, 0, 0, 0, 0, 0, 0, 0, 0, 0, 0, 0, 0, 0, 0, 0, 0, 0, 0, 0, 0, 0, 0, 0, 0, 0, 0, 0, 0, 0, 0, 0, 0, 0, 0, 0, 0, 0, 0, 0, 0, 0, 0, 0, 0, 0, 0, 0, 0, 0, 0, 0, 0, 0, 0, 0, 0, 0, 0, 0, 0, 0, 0, 0, 0, 0, 0, 0, 0, 0]  # GFX
        w28 = u8 0  # SoundTimer
        w29 = u8 0  # DelayTimer
        w30 = u16 0  # StackPointer
        w34 = u16 512  # PC
        w35 = u16 0  # I
        # "GFX - 2048 elemnent U8 Array"
        # "Display - 1 for black, 0 for white"
        # "Input - a 16 bit hex keyboard"
        # "Delay Counters (int)"
        # "Stack with 16 subroutines"
        # "Stack Pointer (int)"
        # "4Kb of Memory"
        # "Program Counter - U16"
        # "Address Pointer I (2 byte - U16)"
        # "16 registers called \"V\""
        # "set most values to 0 and PC to 0x200"
        n13 = for {
          N: 4095 -> [_]
          tunnel: [w46] -> w38 mode=indexing
          w46 = u8 0  # Memory (U8)
        }
        n14 = for {
          N: 15 -> [_]
          tunnel: [w45] -> w36 mode=indexing
          w45 = u8 0  # V (U8)
        }
        n15 = for {
          N: 15 -> [_]
          tunnel: [w44] -> w31 mode=indexing
          w44 = u16 0  # Stack
        }
        n16 = for {
          N: 15 -> [_]
          tunnel: [w40] -> w27 mode=indexing
          w40 = u8 0  # Keys
        }
        n17 = for {
          N: 32 -> [_]
          tunnel: [w41] -> w25 mode=indexing
          n18 = for {
            N: 64 -> [_]
            tunnel: [w43] -> w41 mode=indexing
            w43 = u8 0  # Display
          }
        }
        n19 = Bundle By Name(cluster=w22, "Memory"=w38, "V Registers"=w36, "I"=w35, "PC"=w34, "Stack"=w31, "StackPointer"=w30, "DelayTimer"=w29, "SoundTimer"=w28, "Keys"=w27, "Display"=w25, "GFX"=w24) -> (w23:T2)
      }
      frame "Load ROM & Fontset" {
        # "#future - implement a more graceful rom selection method"
        # "Read the ROM file and load in to memory at PC (should be 0x0200\nfrom the initialization)"
        n20 = call <vilib>:"Application Directory.vi"() -> ("Application Directory"=w55:path)
        n21 = Build Path(base path=w55, name or relative path="ROMs") -> (appended path=w53:path)
        n22 = call "File Dialog"("start path"=w53) -> ("selected path"=w56:path, "cancelled"=w47:bool, "error out"=w49:errorcluster)  [unwired: 11 in, 1 out]
        n23 = case shown="False" w47 {
          tunnel: w58 -> [w61 w75]
          tunnel: [w60 w75] -> w57
          tunnel: w56 -> [w59 _]
          frame False {
            w64 = u8[] [240, 144, 144, 144, 240, 32, 96, 32, 32, 112, 240, 16, 240, 128, 240, 240, 16, 240, 16, 240, 144, 144, 240, 16, 16, 240, 128, 240, 16, 240, 240, 128, 240, 144, 240, 240, 16, 32, 64, 64, 240, 144, 240, 144, 240, 240, 144, 240, 16, 240, 240, 144, 240, 144, 144, 224, 144, 224, 144, 224, 240, 128, 128, 128, 240, 224, 144, 144, 144, 224, 240, 128, 240, 128, 240, 240, 128, 240, 128, 128]  # Chip8 Fontset
            # "Load standard Chip 8\nFontset in at Mem Addr 0"
            n24 = Unbundle By Name(w61) -> ("Memory"=w66:u8[], "PC"=w69:u16)
            n25 = Open/Create/Replace File(file path (use dialog)=w59, access (0:read/write)=enum16{"read/write", "read-only", "write-only"}."read-only") -> (refnum out=w73:refnum<file>)  [unwired: 4 in, 2 out]
            n26 = To Long Integer(number=w69) -> (32bit integer=w67:i32)
            n27 = Read from Binary File(5:u8 0, 10:-1 ("count (1)"), 11:w73) -> (2:w70:u8[], 3:w68:refnum<file>)  [unwired: 3 in, 2 out]
            n28 = Replace Array Subset(array=w66, new element=w70, index=w67) -> (w62:u8[])
            n29 = Close File(refnum=w68) -> ()  [unwired: 1 in, 2 out]
            n30 = Replace Array Subset(array=w62, new element=w64, index=0) -> (w63:u8[])
            n31 = Bundle By Name(cluster=w61, "Memory"=w63) -> (w60:T2)
          }
          frame True {
          }
        }
        n32 = call <vilib>:"Clear Errors.vi"("error in (no error)"=w49, "specific error code to clear (0: all)"=43) -> ()  [unwired: 4 in, 2 out]
        n33 = Select(t=OpcodeEnum."Exit Program", s=w47, f=OpcodeEnum."Fetch Opcode") -> (s? t:f=w50:T1)
      }
      frame "Fetch Opcode", Default {
        # "Get 2 memory addresses at PC and PC+1, then do a conversion\nto U16 and a byte swap on the PC+1 element in order to build\nan Opcode that consists of the 2 U8 values from memory AND'd\ntogether"
        n34 = Unbundle By Name(w89) -> ("Memory"=w87:u8[], "PC"=w90:u16)
        n35 = Increment(x=w90) -> (x+1=w91:u16)
        n36 = To Long Integer(number=w91) -> (32bit integer=w77:i32)
        n37 = To Long Integer(number=w90) -> (32bit integer=w78:i32)
        n38 = Index Array(array=w87, index #1=w78, index #2=w77) -> (element #1=w84:u8, element #2=w76:u8)
        n39 = Type Cast(type=u16 0, x=w76) -> (*(type *) &x=w82:u16)
        n40 = Type Cast(type=u16 0, x=w84) -> (*(type *) &x=w80:u16)
        n41 = Swap Bytes(anything=w82) -> (byte swapped=w79:u16)
        n42 = Or(x=w80, y=w79) -> (x .or. y?=w81:u16)
        n43 = Bundle By Name(cluster=w89, "Opcode"=w81) -> (w88:T2)
      }
      frame "Decode Opcode" {
        # "Grab MSB"
        # "Do several AND functions with various F masks to get most and least significant digits, then logic to determine the appropriate Opcode"
        n44 = Unbundle By Name(w96) -> ("Opcode"=w92:u16)
        n45 = And(x=w92, y=u16 61440) -> (x .and. y?=w94:u16)
        n46 = case shown="0, Default" w94 {
          tunnel: w92 -> [w107 _ _ _ _ _ _ _ w119 _ _ _ _ _ w137 w144]
          tunnel: [w105 OpcodeEnum."1NNN: Jump to Addr NNN" OpcodeEnum."2NNN: Call subroutine at NNN" OpcodeEnum."3XNN: Skip if VX == NN" OpcodeEnum."4XNN: Skip if VX != NN" OpcodeEnum."5XY0: Skip if VX = VY" OpcodeEnum."6XNN: VX = NN" OpcodeEnum."7XNN: Add NN to VX" w117 OpcodeEnum."9XY0: Skip if VX != VY" OpcodeEnum."ANNN: Set I to Addr NNN" OpcodeEnum."BNNN: Jump to Addr NNN + V0" OpcodeEnum."CXNN: Set VX to result of rand" OpcodeEnum."DXYN: Draw Sprite at VX VY" w135 w142] -> w93
          frame 0, Default {
            # "Check LSB"
            n47 = And(x=w107, y=u16 255) -> (x .and. y?=w97:u16)
            n48 = case shown="0, Default" w97 {
              tunnel: [OpcodeEnum."00E0: Clear Display" OpcodeEnum."00EE: Return from subroutine"] -> w98
              frame 0, Default {
                # "Opcode = 00E0: Clear Screen"
              }
              frame 238 {
                # "Opcode = 00EE: Return from subroutine"
              }
            }
            n49 = Not Equal?(x=w97, y=u16 224) -> (x != y?=w102:bool)
            n50 = Not Equal?(x=w97, y=u16 238) -> (x != y?=w101:bool)
            n51 = And(x=w102, y=w101) -> (x .and. y?=w99:bool)
            n52 = Select(t=OpcodeEnum."0NNN: Call", s=w99, f=w98) -> (s? t:f=w105:T1)
          }
          frame 4096 {
            # "1NNN: goto NNN | Jump to address NNN"
          }
          frame 8192 {
            # "2NNN: Calls subroutine at NNN"
          }
          frame 12288 {
            # "3XNN Skips the next instruction if VX == NN (usually the next instruction is a jump to skip a code block"
          }
          frame 16384 {
            # "4XNN: Skips the next instruction if VX doesn't equal NN. (Usually the next instruction is a jump to skip a code block)"
          }
          frame 20480 {
            # "5XY0: Skips the next instruction if VX equals VY. (Usually the next instruction is a jump to skip a code block)"
          }
          frame 24576 {
            # "6XNN: Sets VX to NN"
          }
          frame 28672 {
            # "7XNN: Adds NN to VX (Carry flag is not changed)"
          }
          frame 32768 {
            # "Grab LSB"
            n53 = And(x=w119, y=u16 15) -> (x .and. y?=w118:u16)
            n54 = case shown="E" w118 {
              tunnel: [OpcodeEnum."8XY0: VX = VY" OpcodeEnum."8XY1: VX = VX or VY" OpcodeEnum."8XY2: VX = VX and VY" OpcodeEnum."8XY3: VX = VX xor VY" OpcodeEnum."8XY4: VX += VY" OpcodeEnum."8XY5: VY - VX" OpcodeEnum."8XY6: Sig bit of VX to VF, then shift right" OpcodeEnum."8XY7: Set VX = VY-VX" OpcodeEnum."8XYE: Sig bit of VX to VF, then shift VX left"] -> w117
              frame 0, Default {
              }
              frame 1 {
              }
              frame 2 {
              }
              frame 3 {
              }
              frame 4 {
              }
              frame 5 {
              }
              frame 6 {
              }
              frame 7 {
              }
              frame 14 {
              }
            }
          }
          frame 36864 {
          }
          frame 40960 {
          }
          frame 45056 {
          }
          frame 49152 {
          }
          frame 53248 {
          }
          frame 57344 {
            n55 = And(x=w137, y=u16 255) -> (x .and. y?=w136:u16)
            n56 = case shown="A1" w136 {
              tunnel: [OpcodeEnum."Undefined OpCode" OpcodeEnum."EXA1: Skip if key stored in VX isn't pressed" OpcodeEnum."EX9E: Skip if key stored in VX is pressed"] -> w135
              frame 0, Default {
              }
              frame 161 {
              }
              frame 158 {
              }
            }
          }
          frame 61440 {
            n57 = And(x=w144, y=u16 255) -> (x .and. y?=w143:u16)
            n58 = case shown="7" w143 {
              tunnel: [OpcodeEnum."Undefined OpCode" OpcodeEnum."FX07: Set VX to value of DelayTimer" OpcodeEnum."FX0A: Keypress to VX blocking" OpcodeEnum."FX15: Set Delay Timer to VX" OpcodeEnum."FX18: Set SoundTimer to VX" OpcodeEnum."FX1E: Add VX to I" OpcodeEnum."FX29: Set Loc of Sprite for VX" OpcodeEnum."FX33: Store BCD of VX" OpcodeEnum."FX55: Store V0 to VX" OpcodeEnum."FX65: Fill V0 to VX"] -> w142
              frame 0, Default {
              }
              frame 7 {
              }
              frame 10 {
              }
              frame 21 {
              }
              frame 24 {
              }
              frame 30 {
              }
              frame 41 {
              }
              frame 51 {
              }
              frame 85 {
              }
              frame 101 {
              }
            }
          }
        }
      }
      frame "Update Display" {
        n59 = Unbundle By Name(w159) -> ("Display"=w156:u8[][])
        n60 = call-poly <vilib>:"Draw Unflattened Pixmap.vi"("data"=w156, "color table"=u32[] [16777215, 0, 128, 16711680, 16711935, 8388736, 255, 65535, 65280, 32768, 8388608, 8421376, 12632256, 8421504, 32896, 0]) -> ("new picture"=→"Display":picture)  [unwired: 7 in]
      }
      frame "Exit Program" {
        n61 = property class="App"() -> ("App.Kind"=w161:T3)  [unwired: 2 in, 2 out]
        n62 = case shown="\"Run Time System\"" w161 {
          frame "invalid app kind", Default {
          }
          frame "Development System" {
          }
          frame "Run Time System" {
            n63 = Quit LabVIEW() -> ()  [unwired: 1 in]
          }
        }
      }
      frame "0NNN: Call" {
        # "I haven't really implemented this as it refers to a slightly different chip known as Super Chip 8"
        n64 = Unbundle By Name(w167) -> ("PC"=w169:u16)
        n65 = Increment(x=w169) -> (x+1=w166:u16)
        n66 = Increment(x=w166) -> (x+1=w165:u16)
        n67 = Bundle By Name(cluster=w167, "PC"=w165) -> (w168:T2)
      }
      frame "00E0: Clear Display" {
        # "Fill both Display and GFX with zeros\nthen call Update Display"
        # "// 00E0 - Clear screen\n                case 0x0000:\n                    for (int i = 0; i < 2048; ++i) {\n                        gfx[i] = 0;\n                    }\n                    drawFlag = true;\n                    pc+=2;\n                    break;"
        n68 = Unbundle By Name(w177) -> ("PC"=w179:u16, "Display"=w175:u8[][], "GFX"=w173:u8[])
        n69 = for {
          tunnel: w175 -> [w183] mode=indexing
          tunnel: [w182] -> w174 mode=indexing
          n70 = for {
            tunnel: w183 -> [_] mode=indexing
            tunnel: [u8 0] -> w182 mode=indexing
          }
        }
        n71 = for {
          tunnel: w173 -> [_] mode=indexing
          tunnel: [u8 0] -> w172 mode=indexing
        }
        n72 = Increment(x=w179) -> (x+1=w180:u16)
        n73 = Increment(x=w180) -> (x+1=w176:u16)
        n74 = Bundle By Name(cluster=w177, "PC"=w176, "Display"=w174, "GFX"=w172) -> (w178:T2)
      }
      frame "00EE: Return from subroutine" {
        # "Per cowgod\n00EE - RET\nReturn from a subroutine.\n\nThe interpreter sets the program counter to the address at\n the top of the stack, then subtracts 1 from the stack pointer."
        # "// 00EE - Return from subroutine\n                case 0x000E:\n                    --sp;\n                    pc = stack[sp];\n                    pc += 2;\n                    break;"
        # "not sure if this impliementation is correct- cowgod has a different definition"
        # "pc+=2"
        # "pc=stack[sp]"
        # "--sp"
        # "Return from a stack subroutine and do the proper stack maintainance"
        n75 = Unbundle By Name(w189) -> ("Stack"=w193:u16[], "StackPointer"=w194:u16)
        n76 = Decrement(x=w194) -> (x-1=w185:u16)
        n77 = To Long Integer(number=w185) -> (32bit integer=w186:i32)
        n78 = Index Array(array=w193, index=w186) -> (element=w191:u16)
        n79 = Increment(x=w191) -> (x+1=w192:u16)
        n80 = Increment(x=w192) -> (x+1=w188:u16)
        n81 = Bundle By Name(cluster=w189, "PC"=w188, "StackPointer"=w185) -> (w190:T2)
      }
      frame "1NNN: Jump to Addr NNN" {
        # "// 1NNN - Jumps to address NNN\n        case 0x1000:\n            pc = opcode & 0x0FFF;\n            break;"
        # "Set PC to address NNN"
        n82 = Unbundle By Name(w198) -> ("Opcode"=w200:u16)
        n83 = And(x=w200, y=u16 4095) -> (x .and. y?=w196:u16)
        n84 = Bundle By Name(cluster=w198, "PC"=w196) -> (w197:T2)
      }
      frame "2NNN: Call subroutine at NNN" {
        # "// 2NNN - Calls subroutine at NNN\n        case 0x2000:\n            stack[sp] = pc;\n            ++sp;\n            pc = opcode & 0x0FFF;\n            break;"
        # "This opcode calls the subroutine at address NNN. Because we \nwill need to temporary jump to address NNN, it means that we\n should store the current address of the program counter in the \nstack. After storing the value of the program counter in the stack, \nincrease the stack pointer to prevent overwriting the current \nstack. Now that we have stored the program counter, we can \nset it to the address NNN. Remember, because we’re calling a\nsubroutine at a specific address, you should not increase the \nprogram counter by two."
        # "pc = opcode & 0x0FFF"
        # "sp++;"
        # "stack[sp] = pc;"
        n85 = Unbundle By Name(w205) -> ("Opcode"=w212:u16, "Stack"=w209:u16[], "StackPointer"=w207:u16, "PC"=w208:u16)
        n86 = And(x=u16 4095 ("y"), y=w212) -> (x .and. y?=w204:u16)
        n87 = To Long Integer(number=w207) -> (32bit integer=w202:i32)
        n88 = Replace Array Subset(array=w209, new element=w208, index=w202) -> (w201:u16[])
        n89 = Increment(x=w207) -> (x+1=w203:u16)
        n90 = Bundle By Name(cluster=w205, "PC"=w204, "StackPointer"=w203, "Stack"=w201) -> (w206:T2)
      }
      frame "3XNN: Skip if VX == NN" {
        # "// 3XNN - Skips the next instruction if VX equals NN.\n        case 0x3000:\n            if (V[(opcode & 0x0F00) >> 8] == (opcode & 0x00FF))\n                pc += 4;\n            else\n                pc += 2;\n            break;"
        n91 = Unbundle By Name(w226) -> ("PC"=w220:u16, "Opcode"=w218:u16, "V Registers"=w224:u8[])
        n92 = call "Opcode at X.vi"("X Position"=enum16{"First", "Second", "Third", "Fourth"}."Second", "Opcode"=w218) -> ("Opcode at X Position (U8)"=w223:u8)  [unwired: 9 in]
        n93 = To Long Integer(number=w223) -> (32bit integer=w217:i32)
        n94 = call "Opcode at last 2 positions.vi"("Opcode"=w218) -> ("00FF"=w221:u8)  [unwired: 10 in]
        n95 = Index Array(array=w224, index=w217) -> (element=w222:u8)
        n96 = Equal?(x=w221, y=w222) -> (x = y?=w216:bool)
        n97 = Select(t=u16 4 ("y"), s=w216, f=u16 2 ("y")) -> (s? t:f=w213:u16)
        n98 = Add(x=w220, y=w213) -> (x+y=w219:u16)
        n99 = Bundle By Name(cluster=w226, "PC"=w219) -> (w227:T2)
      }
      frame "4XNN: Skip if VX != NN" {
        # "// 4XNN - Skips the next instruction if VX does not equal NN.\n        case 0x4000:\n            if (V[(opcode & 0x0F00) >> 8] != (opcode & 0x00FF))\n                pc += 4;\n            else\n                pc += 2;\n            break;"
        n100 = Unbundle By Name(w235) -> ("PC"=w239:u16, "Opcode"=w237:u16, "V Registers"=w243:u8[])
        n101 = call "Opcode at X.vi"("X Position"=enum16{"First", "Second", "Third", "Fourth"}."Second", "Opcode"=w237) -> ("Opcode at X Position (U8)"=w242:u8)  [unwired: 9 in]
        n102 = To Long Integer(number=w242) -> (32bit integer=w236:i32)
        n103 = call "Opcode at last 2 positions.vi"("Opcode"=w237) -> ("00FF"=w240:u8)  [unwired: 10 in]
        n104 = Index Array(array=w243, index=w236) -> (element=w241:u8)
        n105 = Not Equal?(x=w240, y=w241) -> (x != y?=w230:bool)
        n106 = Select(t=u16 4 ("y"), s=w230, f=u16 2 ("y")) -> (s? t:f=w229:u16)
        n107 = Add(x=w239, y=w229) -> (x+y=w238:u16)
        n108 = Bundle By Name(cluster=w235, "PC"=w238) -> (w233:T2)
      }
      frame "5XY0: Skip if VX = VY" {
        # "// 5XY0 - Skips the next instruction if VX equals VY.\n        case 0x5000:\n            if (V[(opcode & 0x0F00) >> 8] == V[(opcode & 0x00F0) >> 4])\n                pc += 4;\n            else\n                pc += 2;\n            break;"
        n109 = Unbundle By Name(w259) -> ("PC"=w261:u16, "V Registers"=w245:u8[], "Opcode"=w257:u16)
        n110 = call "Opcode at X.vi"("X Position"=enum16{"First", "Second", "Third", "Fourth"}."Second", "Opcode"=w257) -> ("Opcode at X Position (U8)"=w254:u8)  [unwired: 9 in]
        n111 = call "Opcode at X.vi"("X Position"=enum16{"First", "Second", "Third", "Fourth"}."Third", "Opcode"=w257) -> ("Opcode at X Position (U8)"=w262:u8)  [unwired: 9 in]
        n112 = To Long Integer(number=w254) -> (32bit integer=w255:i32)
        n113 = To Long Integer(number=w262) -> (32bit integer=w247:i32)
        n114 = Index Array(array=w245, index #1=w255, index #2=w247) -> (element #1=w253:u8, element #2=w246:u8)
        n115 = Equal?(x=w253, y=w246) -> (x = y?=w248:bool)
        n116 = Select(t=u16 4 ("y"), s=w248, f=u16 2 ("y")) -> (s? t:f=w249:u16)
        n117 = Add(x=w261, y=w249) -> (x+y=w260:u16)
        n118 = Bundle By Name(cluster=w259, "PC"=w260) -> (w258:T2)
      }
      frame "6XNN: VX = NN" {
        # "// 6XNN - Sets VX to NN.\n        case 0x6000:\n            V[(opcode & 0x0F00) >> 8] = opcode & 0x00FF;\n            pc += 2;\n            break;"
        # "Take the second nibble (X) and use it to index the V registers, then define that value as NN"
        n119 = Unbundle By Name(w275) -> ("V Registers"=w264:u8[], "Opcode"=w266:u16, "PC"=w272:u16)
        n120 = Increment(x=w272) -> (x+1=w271:u16)
        n121 = call "Opcode at X.vi"("X Position"=enum16{"First", "Second", "Third", "Fourth"}."Second", "Opcode"=w266) -> ("Opcode at X Position (U8)"=w267:u8)  [unwired: 9 in]
        n122 = call "Opcode at last 2 positions.vi"("Opcode"=w266) -> ("00FF"=w265:u8)  [unwired: 10 in]
        n123 = Increment(x=w271) -> (x+1=w270:u16)
        n124 = To Long Integer(number=w267) -> (32bit integer=w269:i32)
        n125 = Replace Array Subset(array=w264, new element=w265, index=w269) -> (w274:u8[])
        n126 = Bundle By Name(cluster=w275, "V Registers"=w274, "PC"=w270) -> (w276:T2)
      }
      frame "7XNN: Add NN to VX" {
        # "// 7XNN - Adds NN to VX.\n        case 0x7000:\n            V[(opcode & 0x0F00) >> 8] += opcode & 0x00FF;\n            pc += 2;\n            break;"
        # "Get NN"
        # "Get X"
        # "Adds NN to VX. (Carry flag is not changed)"
        n127 = Unbundle By Name(w285) -> ("PC"=w282:u16, "V Registers"=w287:u8[], "Opcode"=w277:u16)
        n128 = call "Opcode at X.vi"("X Position"=enum16{"First", "Second", "Third", "Fourth"}."Second", "Opcode"=w277) -> ("Opcode at X Position (U8)"=w279:u8)  [unwired: 9 in]
        n129 = call "Opcode at last 2 positions.vi"("Opcode"=w277) -> ("00FF"=w278:u8)  [unwired: 10 in]
        n130 = Equal?(x=w279, y=u8 15) -> (x = y?=w289:bool)
        n131 = case shown="False" w289 {
          tunnel: w287 -> [w295 w299]
          tunnel: w279 -> [w294 _]
          tunnel: w278 -> [w293 _]
          tunnel: [w292 w299] -> w284
          frame False {
            n132 = To Long Integer(number=w294) -> (32bit integer=w291:i32)
            n133 = in-place {
              in-place-border: w293 -> [w298]
              n134 = in-place-array #1(w295, w291) -> (w297:u8)
              n135 = Add(x=w298, y=w297) -> (x+y=w296:u8)
              n136 = in-place-array #1(w296) -> (w292:u8[])  [unwired: 1 out]
            }
          }
          frame True {
            # "Carry flag (VF) is not changed"
          }
        }
        n137 = Increment(x=w282) -> (x+1=w283:u16)
        n138 = Increment(x=w283) -> (x+1=w281:u16)
        n139 = Bundle By Name(cluster=w285, "PC"=w281, "V Registers"=w284) -> (w286:T2)
      }
      frame "8XY0: VX = VY" {
        # "// 8XY0 - Sets VX to the value of VY.\n                case 0x0000:\n                    V[(opcode & 0x0F00) >> 8] = V[(opcode & 0x00F0) >> 4];\n                    pc += 2;\n                    break;"
        # "VX"
        # "VY"
        n140 = Unbundle By Name(w308) -> ("PC"=w305:u16, "V Registers"=w312:u8[], "Opcode"=w300:u16)
        n141 = call "Opcode at X.vi"("X Position"=enum16{"First", "Second", "Third", "Fourth"}."Second", "Opcode"=w300) -> ("Opcode at X Position (U8)"=w311:u8)  [unwired: 9 in]
        n142 = call "Opcode at X.vi"("X Position"=enum16{"First", "Second", "Third", "Fourth"}."Third", "Opcode"=w300) -> ("Opcode at X Position (U8)"=w310:u8)  [unwired: 9 in]
        n143 = Increment(x=w305) -> (x+1=w306:u16)
        n144 = To Long Integer(number=w311) -> (32bit integer=w301:i32)
        n145 = To Long Integer(number=w310) -> (32bit integer=w302:i32)
        n146 = Increment(x=w306) -> (x+1=w304:u16)
        n147 = in-place {
          n148 = in-place-array #2(w312, w301, w302) -> (w315:u8)  [unwired: 1 out]
          n149 = in-place-array #2(w315, w315) -> (w303:u8[])  [unwired: 2 out]
        }
        n150 = Bundle By Name(cluster=w308, "PC"=w304, "V Registers"=w303) -> (w309:T2)
      }
      frame "8XY1: VX = VX or VY" {
        # "// 8XY1 - Sets VX to (VX OR VY).\n                case 0x0001:\n                    V[(opcode & 0x0F00) >> 8] |= V[(opcode & 0x00F0) >> 4];\n                    pc += 2;\n                    break;"
        n151 = Unbundle By Name(w328) -> ("PC"=w329:u16, "V Registers"=w322:u8[], "Opcode"=w316:u16)
        n152 = call "Opcode at X.vi"("X Position"=enum16{"First", "Second", "Third", "Fourth"}."Second", "Opcode"=w316) -> ("Opcode at X Position (U8)"=w321:u8)  [unwired: 9 in]
        n153 = call "Opcode at X.vi"("X Position"=enum16{"First", "Second", "Third", "Fourth"}."Third", "Opcode"=w316) -> ("Opcode at X Position (U8)"=w323:u8)  [unwired: 9 in]
        n154 = To Long Integer(number=w321) -> (32bit integer=w320:i32)
        n155 = To Long Integer(number=w323) -> (32bit integer=w317:i32)
        n156 = in-place {
          n157 = in-place-array #3(w322, w320, w317) -> (w331:u8, w332:u8)
          n158 = Or(x=w331, y=w332) -> (x .or. y?=w333:u8)
          n159 = in-place-array #3(w333, w332) -> (w319:u8[])  [unwired: 2 out]
        }
        n160 = Increment(x=w329) -> (x+1=w330:u16)
        n161 = Increment(x=w330) -> (x+1=w326:u16)
        n162 = Bundle By Name(cluster=w328, "PC"=w326, "V Registers"=w319) -> (w327:T2)
      }
      frame "8XY2: VX = VX and VY" {
        # "// 8XY2 - Sets VX to (VX AND VY).\n                case 0x0002:\n                    V[(opcode & 0x0F00) >> 8] &= V[(opcode & 0x00F0) >> 4];\n                    pc += 2;\n                    break;"
        n163 = Unbundle By Name(w338) -> ("PC"=w347:u16, "V Registers"=w342:u8[], "Opcode"=w334:u16)
        n164 = call "Opcode at X.vi"("X Position"=enum16{"First", "Second", "Third", "Fourth"}."Second", "Opcode"=w334) -> ("Opcode at X Position (U8)"=w341:u8)  [unwired: 9 in]
        n165 = call "Opcode at X.vi"("X Position"=enum16{"First", "Second", "Third", "Fourth"}."Third", "Opcode"=w334) -> ("Opcode at X Position (U8)"=w343:u8)  [unwired: 9 in]
        n166 = To Long Integer(number=w341) -> (32bit integer=w340:i32)
        n167 = To Long Integer(number=w343) -> (32bit integer=w335:i32)
        n168 = in-place {
          n169 = in-place-array #4(w342, w340, w335) -> (w351:u8, w349:u8)
          n170 = And(x=w351, y=w349) -> (x .and. y?=w350:u8)
          n171 = in-place-array #4(w350, w349) -> (w339:u8[])  [unwired: 2 out]
        }
        n172 = Increment(x=w347) -> (x+1=w348:u16)
        n173 = Increment(x=w348) -> (x+1=w346:u16)
        n174 = Bundle By Name(cluster=w338, "PC"=w346, "V Registers"=w339) -> (w337:T2)
      }
      frame "8XY3: VX = VX xor VY" {
        # "// 8XY3 - Sets VX to (VX XOR VY).\n                case 0x0003:\n                    V[(opcode & 0x0F00) >> 8] ^= V[(opcode & 0x00F0) >> 4];\n                    pc += 2;\n                    break;"
        n175 = Unbundle By Name(w354) -> ("PC"=w365:u16, "V Registers"=w360:u8[], "Opcode"=w352:u16)
        n176 = call "Opcode at X.vi"("X Position"=enum16{"First", "Second", "Third", "Fourth"}."Second", "Opcode"=w352) -> ("Opcode at X Position (U8)"=w359:u8)  [unwired: 9 in]
        n177 = call "Opcode at X.vi"("X Position"=enum16{"First", "Second", "Third", "Fourth"}."Third", "Opcode"=w352) -> ("Opcode at X Position (U8)"=w361:u8)  [unwired: 9 in]
        n178 = To Long Integer(number=w359) -> (32bit integer=w358:i32)
        n179 = To Long Integer(number=w361) -> (32bit integer=w353:i32)
        n180 = in-place {
          n181 = in-place-array #5(w360, w358, w353) -> (w369:u8, w367:u8)
          n182 = Exclusive Or(1:w367, 2:w369) -> (0:w368:u8)
          n183 = in-place-array #5(w368, w367) -> (w357:u8[])  [unwired: 2 out]
        }
        n184 = Increment(x=w365) -> (x+1=w366:u16)
        n185 = Increment(x=w366) -> (x+1=w364:u16)
        n186 = Bundle By Name(cluster=w354, "PC"=w364, "V Registers"=w357) -> (w355:T2)
      }
      frame "8XY4: VX += VY" {
        # "// 8XY4 - Adds VY to VX. VF is set to 1 when there's a carry,\n                // and to 0 when there isn't.\n                case 0x0004:\n                    V[(opcode & 0x0F00) >> 8] += V[(opcode & 0x00F0) >> 4];\n                    if(V[(opcode & 0x00F0) >> 4] > (0xFF - V[(opcode & 0x0F00) >> 8]))\n                        V[0xF] = 1; //carry\n                    else\n                        V[0xF] = 0;\n                    pc += 2;\n                    break;"
        # "Adds VY to VX. VF is set to 1 when there's a carry, and to 0 when there isn't."
        n187 = Unbundle By Name(w384) -> ("PC"=w383:u16, "V Registers"=w373:u8[], "Opcode"=w380:u16)
        n188 = call "Opcode at X.vi"("X Position"=enum16{"First", "Second", "Third", "Fourth"}."Second", "Opcode"=w380) -> ("Opcode at X Position (U8)"=w376:u8)  [unwired: 9 in]
        n189 = call "Opcode at X.vi"("X Position"=enum16{"First", "Second", "Third", "Fourth"}."Third", "Opcode"=w380) -> ("Opcode at X Position (U8)"=w377:u8)  [unwired: 9 in]
        n190 = To Long Integer(number=15) -> (32bit integer=w370:i32)
        n191 = To Long Integer(number=w376) -> (32bit integer=w375:i32)
        n192 = To Long Integer(number=w377) -> (32bit integer=w371:i32)
        n193 = in-place {
          n194 = in-place-array #6(w373, w375, w371, w370) -> (w392:u8, w387:u8)  [unwired: 1 out]
          n195 = Add(x=w392, y=w387) -> (x+y=w393:u8)
          n196 = Greater?(x=w387, y=w392) -> (0:w391:bool)
          n197 = Select(t=u8 1, s=w391, f=u8 0) -> (s? t:f=w388:u8)
          n198 = in-place-array #6(w393, w387, w388) -> (w374:u8[])  [unwired: 3 out]
        }
        n199 = Increment(x=w383) -> (x+1=w382:u16)
        n200 = Increment(x=w382) -> (x+1=w381:u16)
        n201 = Bundle By Name(cluster=w384, "PC"=w381, "V Registers"=w374) -> (w385:T2)
      }
      frame "8XY5: VY - VX" {
        # "// 8XY5 - VY is subtracted from VX. VF is set to 0 when\n                // there's a borrow, and 1 when there isn't.\n                case 0x0005:\n                    if(V[(opcode & 0x00F0) >> 4] > V[(opcode & 0x0F00) >> 8])\n                        V[0xF] = 0; // there is a borrow\n                    else\n                        V[0xF] = 1;\n                    V[(opcode & 0x0F00) >> 8] -= V[(opcode & 0x00F0) >> 4];\n                    pc += 2;\n                    break;"
        n202 = Unbundle By Name(w402) -> ("PC"=w410:u16, "V Registers"=w399:u8[], "Opcode"=w407:u16)
        n203 = call "Opcode at X.vi"("X Position"=enum16{"First", "Second", "Third", "Fourth"}."Second", "Opcode"=w407) -> ("Opcode at X Position (U8)"=w403:u8)  [unwired: 9 in]
        n204 = call "Opcode at X.vi"("X Position"=enum16{"First", "Second", "Third", "Fourth"}."Third", "Opcode"=w407) -> ("Opcode at X Position (U8)"=w404:u8)  [unwired: 9 in]
        n205 = To Long Integer(number=15) -> (32bit integer=w394:i32)
        n206 = To Long Integer(number=w403) -> (32bit integer=w398:i32)
        n207 = To Long Integer(number=w404) -> (32bit integer=w395:i32)
        n208 = in-place {
          n209 = in-place-array #7(w399, w398, w395, w394) -> (w416:u8, w411:u8)  [unwired: 1 out]
          n210 = Subtract(x=w416, y=w411) -> (x-y=w417:u8)
          n211 = Greater?(x=w411, y=w416) -> (0:w415:bool)
          n212 = Select(t=u8 0, s=w415, f=u8 1) -> (s? t:f=w412:u8)
          n213 = in-place-array #7(w417, w411, w412) -> (w396:u8[])  [unwired: 3 out]
        }
        n214 = Increment(x=w410) -> (x+1=w409:u16)
        n215 = Increment(x=w409) -> (x+1=w408:u16)
        n216 = Bundle By Name(cluster=w402, "PC"=w408, "V Registers"=w396) -> (w401:T2)
      }
      frame "8XY6: Sig bit of VX to VF, then shift right" {
        # "this may be a buggy interpretation of the opcode intention"
        # "// 0x8XY6 - Shifts VX right by one. VF is set to the value of\n                // the least significant bit of VX before the shift.\n                case 0x0006:\n                    V[0xF] = V[(opcode & 0x0F00) >> 8] & 0x1;\n                    V[(opcode & 0x0F00) >> 8] >>= 1;\n                    pc += 2;\n                    break;"
        # "#NOTSURE ABOUT THIS ONE could be the source of some of the bugs"
        n217 = Unbundle By Name(w423) -> ("PC"=w419:u16, "V Registers"=w428:u8[], "Opcode"=w430:u16)
        n218 = call "Opcode at X.vi"("X Position"=enum16{"First", "Second", "Third", "Fourth"}."Second", "Opcode"=w430) -> ("Opcode at X Position (U8)"=w427:u8)  [unwired: 9 in]
        n219 = To Long Integer(number=u8 15 ("y")) -> (32bit integer=w424:i32)
        n220 = To Long Integer(number=w427) -> (32bit integer=w426:i32)
        n221 = in-place {
          n222 = in-place-array #8(w428, w424, w426) -> (w435:u8)  [unwired: 1 out]
          n223 = Negate(x=i8 1 ("y")) -> (-x=w434:i8)
          n224 = Logical Shift(y=w434, x=w435) -> (x << y=w432:u8)
          n225 = And(x=w435, y=u8 1) -> (x .and. y?=w436:u8)
          n226 = in-place-array #8(w436, w432) -> (w421:u8[])  [unwired: 2 out]
        }
        n227 = Increment(x=w419) -> (x+1=w420:u16)
        n228 = Increment(x=w420) -> (x+1=w418:u16)
        n229 = Bundle By Name(cluster=w423, "PC"=w418, "V Registers"=w421) -> (w422:T2)
      }
      frame "8XY7: Set VX = VY-VX" {
        # "// 0x8XY7: Sets VX to VY minus VX. VF is set to 0 when there's\n                // a borrow, and 1 when there isn't.\n                case 0x0007:\n                    if(V[(opcode & 0x0F00) >> 8] > V[(opcode & 0x00F0) >> 4])\t// VY-VX\n                        V[0xF] = 0; // there is a borrow\n                    else\n                        V[0xF] = 1;\n                    V[(opcode & 0x0F00) >> 8] = V[(opcode & 0x00F0) >> 4] - V[(opcode & 0x0F00) >> 8];\n                    pc += 2;\n                    break;"
        n230 = Unbundle By Name(w453) -> ("PC"=w447:u16, "V Registers"=w449:u8[], "Opcode"=w452:u16)
        n231 = call "Opcode at X.vi"("X Position"=enum16{"First", "Second", "Third", "Fourth"}."Second", "Opcode"=w452) -> ("Opcode at X Position (U8)"=w445:u8)  [unwired: 9 in]
        n232 = call "Opcode at X.vi"("X Position"=enum16{"First", "Second", "Third", "Fourth"}."Third", "Opcode"=w452) -> ("Opcode at X Position (U8)"=w444:u8)  [unwired: 9 in]
        n233 = To Long Integer(number=15) -> (32bit integer=w440:i32)
        n234 = To Long Integer(number=w445) -> (32bit integer=w443:i32)
        n235 = To Long Integer(number=w444) -> (32bit integer=w442:i32)
        n236 = in-place {
          n237 = in-place-array #9(w449, w443, w442, w440) -> (w457:u8, w455:u8)  [unwired: 1 out]
          n238 = Subtract(x=w455, y=w457) -> (x-y=w456:u8)
          n239 = Greater?(x=w457, y=w455) -> (0:w461:bool)
          n240 = Select(t=u8 1, s=w461, f=u8 0) -> (s? t:f=w458:u8)
          n241 = in-place-array #9(w456, w455, w458) -> (w439:u8[])  [unwired: 3 out]
        }
        n242 = Increment(x=w447) -> (x+1=w448:u16)
        n243 = Increment(x=w448) -> (x+1=w446:u16)
        n244 = Bundle By Name(cluster=w453, "PC"=w446, "V Registers"=w439) -> (w454:T2)
      }
      frame "8XYE: Sig bit of VX to VF, then shift VX left" {
        # "// 0x8XYE: Shifts VX left by one. VF is set to the value of\n                // the most significant bit of VX before the shift.\n                case 0x000E:\n                    V[0xF] = V[(opcode & 0x0F00) >> 8] >> 7;\n                    V[(opcode & 0x0F00) >> 8] <<= 1;\n                    pc += 2;\n                    break;"
        # "#notsure on this one either - need to double check with debugging and insertion"
        n245 = Unbundle By Name(w474) -> ("PC"=w471:u16, "V Registers"=w467:u8[], "Opcode"=w469:u16)
        n246 = call "Opcode at X.vi"("X Position"=enum16{"First", "Second", "Third", "Fourth"}."Second", "Opcode"=w469) -> ("Opcode at X Position (U8)"=w464:u8)  [unwired: 9 in]
        n247 = To Long Integer(number=u8 15) -> (32bit integer=w465:i32)
        n248 = To Long Integer(number=w464) -> (32bit integer=w463:i32)
        n249 = in-place {
          n250 = in-place-array #10(w467, w465, w463) -> (w478:u8)  [unwired: 1 out]
          n251 = Logical Shift(y=i16 1, x=w478) -> (x << y=w476:u8)
          n252 = Logical Shift(y=i16 -7, x=w478) -> (x << y=w479:u8)
          n253 = in-place-array #10(w479, w476) -> (w462:u8[])  [unwired: 2 out]
        }
        n254 = Increment(x=w471) -> (x+1=w472:u16)
        n255 = Increment(x=w472) -> (x+1=w470:u16)
        n256 = Bundle By Name(cluster=w474, "PC"=w470, "V Registers"=w462) -> (w473:T2)
      }
      frame "9XY0: Skip if VX != VY" {
        # "// 9XY0 - Skips the next instruction if VX doesn't equal VY.\n        case 0x9000:\n            if (V[(opcode & 0x0F00) >> 8] != V[(opcode & 0x00F0) >> 4])\n                pc += 4;\n            else\n                pc += 2;\n            break;"
        n257 = Unbundle By Name(w495) -> ("PC"=w497:u16, "V Registers"=w489:u8[], "Opcode"=w483:u16)
        n258 = call "Opcode at X.vi"("X Position"=enum16{"First", "Second", "Third", "Fourth"}."Second", "Opcode"=w483) -> ("Opcode at X Position (U8)"=w490:u8)  [unwired: 9 in]
        n259 = call "Opcode at X.vi"("X Position"=enum16{"First", "Second", "Third", "Fourth"}."Third", "Opcode"=w483) -> ("Opcode at X Position (U8)"=w498:u8)  [unwired: 9 in]
        n260 = To Long Integer(number=w490) -> (32bit integer=w491:i32)
        n261 = To Long Integer(number=w498) -> (32bit integer=w482:i32)
        n262 = Index Array(array=w489, index #1=w491, index #2=w482) -> (element #1=w488:u8, element #2=w481:u8)
        n263 = Not Equal?(x=w488, y=w481) -> (x != y?=w485:bool)
        n264 = Select(t=u16 4 ("y"), s=w485, f=u16 2 ("y")) -> (s? t:f=w484:u16)
        n265 = Add(x=w497, y=w484) -> (x+y=w496:u16)
        n266 = Bundle By Name(cluster=w495, "PC"=w496) -> (w494:T2)
      }
      frame "ANNN: Set I to Addr NNN" {
        # "// ANNN - Sets I to the address NNN.\n        case 0xA000:\n            I = opcode & 0x0FFF;\n            pc += 2;\n            break;"
        n267 = Unbundle By Name(w507) -> ("Opcode"=w500:u16, "PC"=w504:u16)
        n268 = Increment(x=w504) -> (x+1=w505:u16)
        n269 = Increment(x=w505) -> (x+1=w502:u16)
        n270 = And(x=u16 4095 ("y"), y=w500) -> (x .and. y?=w506:u16)
        n271 = Bundle By Name(cluster=w507, "I"=w506, "PC"=w502) -> (w508:T2)
      }
      frame "BNNN: Jump to Addr NNN + V0" {
        # "// BNNN - Jumps to the address NNN plus V0.\n        case 0xB000:\n            pc = (opcode & 0x0FFF) + V[0];\n            break;"
        n272 = Unbundle By Name(w511) -> ("V Registers"=w517:u8[], "Opcode"=w519:u16)
        n273 = Index Array(array=w517, index=0) -> (element=w515:u8)
        n274 = And(x=w519, y=u16 4095) -> (x .and. y?=w514:u16)
        n275 = To Unsigned Word Integer(number=w515) -> (unsigned 16bit integer=w513:u16)
        n276 = Add(x=w513, y=w514) -> (x+y=w510:u16)
        n277 = Bundle By Name(cluster=w511, "PC"=w510) -> (w512:T2)
      }
      frame "CXNN: Set VX to result of rand" {
        # "// CXNN - Sets VX to a random number, masked by NN.\n        case 0xC000:\n            V[(opcode & 0x0F00) >> 8] = (rand() % (0xFF + 1)) & (opcode & 0x00FF);\n            pc += 2;\n            break;"
        n278 = Unbundle By Name(w530) -> ("PC"=w529:u16, "V Registers"=w524:u8[], "Opcode"=w525:u16)
        n279 = call "Opcode at X.vi"("X Position"=enum16{"First", "Second", "Third", "Fourth"}."Second", "Opcode"=w525) -> ("Opcode at X Position (U8)"=w523:u8)  [unwired: 9 in]
        n280 = call "Opcode at last 2 positions.vi"("Opcode"=w525) -> ("00FF"=w521:u8)  [unwired: 10 in]
        n281 = To Long Integer(number=w523) -> (32bit integer=w522:i32)
        n282 = in-place {
          in-place-border: w521 -> [w538]
          n283 = in-place-array #11(w524, w522) -> ()  [unwired: 1 out]
          n284 = Random Number (0-1)() -> (number: 0 to 1=w540:dbl)
          n285 = Multiply(x=w540, y=255.0) -> (x*y=w535:dbl)
          n286 = Quotient & Remainder(x=w535, y=1.0) -> (floor(x/y)=w533:dbl)  [unwired: 1 out]
          n287 = To Unsigned Byte Integer(number=w533) -> (unsigned 8bit integer=w537:u8)
          n288 = And(x=w538, y=w537) -> (x .and. y?=w536:u8)
          n289 = in-place-array #11(w536) -> (w520:u8[])  [unwired: 1 out]
        }
        n290 = Increment(x=w529) -> (x+1=w528:u16)
        n291 = Increment(x=w528) -> (x+1=w527:u16)
        n292 = Bundle By Name(cluster=w530, "PC"=w527, "V Registers"=w520) -> (w531:T2)
      }
      frame "DXYN: Draw Sprite at VX VY" {
        # "For collision detection set VF to 0 before doing Draw"
        n293 = Unbundle By Name(w546) -> ("V Registers"=w545:u8[])
        n294 = To Long Integer(number=u8 15) -> (32bit integer=w543:i32)
        n295 = Replace Array Subset(array=w545, new element=u8 0 ("new element/subarray"), index=w543) -> (w541:u8[])
        n296 = Bundle By Name(cluster=w546, "V Registers"=w541) -> (w547:T2)
        n297 = call "DXYN.vi"("Variables and Memory in"=w547) -> ("Variables and Memory out"=w548:T2)  [unwired: 10 in]
      }
      frame "EX9E: Skip if key stored in VX is pressed" {
        # "// EX9E - Skips the next instruction if the key stored\n                // in VX is pressed.\n                case 0x009E:\n                    if (key[V[(opcode & 0x0F00) >> 8]] != 0)\n                        pc +=  4;\n                    else\n                        pc += 2;\n                    break;"
        n298 = Unbundle By Name(w557) -> ("PC"=w568:u16, "Keys"=w565:u8[], "V Registers"=w566:u8[], "Opcode"=w551:u16)
        n299 = call "Opcode at X.vi"("X Position"=enum16{"First", "Second", "Third", "Fourth"}."Second", "Opcode"=w551) -> ("Opcode at X Position (U8)"=w559:u8)  [unwired: 9 in]
        n300 = To Long Integer(number=w559) -> (32bit integer=w560:i32)
        n301 = Index Array(array=w566, index=w560) -> (element=w562:u8)
        n302 = To Long Integer(number=w562) -> (32bit integer=w561:i32)
        n303 = Index Array(array=w565, index=w561) -> (element=w564:u8)
        n304 = Equal To 0?(x=w564) -> (x = 0?=w563:bool)
        n305 = Not(x=w563) -> (.not. x?=w553:bool)
        n306 = Select(t=u16 4 ("y"), s=w553, f=u16 2 ("y")) -> (s? t:f=w552:u16)
        n307 = Add(x=w568, y=w552) -> (x+y=w567:u16)
        n308 = Bundle By Name(cluster=w557, "PC"=w567) -> (w558:T2)
      }
      frame "EXA1: Skip if key stored in VX isn't pressed" {
        # "// EXA1 - Skips the next instruction if the key stored\n                // in VX isn't pressed.\n                case 0x00A1:\n                    if (key[V[(opcode & 0x0F00) >> 8]] == 0)\n                        pc +=  4;\n                    else\n                        pc += 2;\n                    break;"
        n309 = Unbundle By Name(w585) -> ("PC"=w586:u16, "Keys"=w580:u8[], "V Registers"=w581:u8[], "Opcode"=w570:u16)
        n310 = call "Opcode at X.vi"("X Position"=enum16{"First", "Second", "Third", "Fourth"}."Second", "Opcode"=w570) -> ("Opcode at X Position (U8)"=w575:u8)  [unwired: 9 in]
        n311 = To Long Integer(number=w575) -> (32bit integer=w576:i32)
        n312 = Index Array(array=w581, index=w576) -> (element=w578:u8)
        n313 = To Long Integer(number=w578) -> (32bit integer=w577:i32)
        n314 = Index Array(array=w580, index=w577) -> (element=w579:u8)
        n315 = Equal To 0?(x=w579) -> (x = 0?=w572:bool)
        n316 = Select(t=u16 4 ("y"), s=w572, f=u16 2 ("y")) -> (s? t:f=w571:u16)
        n317 = Add(x=w586, y=w571) -> (x+y=w583:u16)
        n318 = Bundle By Name(cluster=w585, "PC"=w583) -> (w584:T2)
      }
      frame "FX07: Set VX to value of DelayTimer" {
        # "// FX07 - Sets VX to the value of the delay timer\n                case 0x0007:\n                    V[(opcode & 0x0F00) >> 8] = delay_timer;\n                    pc += 2;\n                    break;"
        n319 = Unbundle By Name(w599) -> ("PC"=w598:u16, "V Registers"=w595:u8[], "Opcode"=w594:u16, "DelayTimer"=w591:u8)
        n320 = Increment(x=w598) -> (x+1=w597:u16)
        n321 = call "Opcode at X.vi"("X Position"=enum16{"First", "Second", "Third", "Fourth"}."Second", "Opcode"=w594) -> ("Opcode at X Position (U8)"=w593:u8)  [unwired: 9 in]
        n322 = Increment(x=w597) -> (x+1=w596:u16)
        n323 = To Long Integer(number=w593) -> (32bit integer=w590:i32)
        n324 = Replace Array Subset(array=w595, new element=w591, index=w590) -> (w589:u8[])
        n325 = Bundle By Name(cluster=w599, "PC"=w596, "V Registers"=w589) -> (w600:T2)
      }
      frame "FX0A: Keypress to VX blocking" {
        # "reimplemented the key get code here, a bit sloppy, but it works"
        # "// FX0A - A key press is awaited, and then stored in VX\n                case 0x000A:\n                {\n                    bool key_pressed = false;\n\n                    for(int i = 0; i < 16; ++i)\n                    {\n                        if(key[i] != 0)\n                        {\n                            V[(opcode & 0x0F00) >> 8] = i;\n                            key_pressed = true;\n                        }\n                    }\n\n                    // If no key is pressed, return and try again.\n                    if(!key_pressed)\n                        return;\n\n                    pc += 2;\n                }\n                    break;"
        n326 = while {
          tunnel: [w616] -> w601
          stop <- w617 stop-if-true
          n327 = event shown="[0] Key Up" {
            selector: _ -> [_ _]
            dyn-events: _ -> [_ _]
            timeout: _ -> [_ _]
            tunnel: [u8[] [0, 0, 0, 0, 0, 0, 0, 0, 0, 0, 0, 0, 0, 0, 0, 0] ("Keys") w619] -> w615
            event Key Up {
              n328 = event-data() -> ()  [unwired: 1 in, 1 out]
            }
            event Key Down {
              n329 = event-data() -> ("Char"=w620:i16)  [unwired: 1 in]
              n330 = case shown="78" w620 {
                tunnel: [u8[] [0, 0, 0, 0, 0, 0, 0, 0, 0, 0, 0, 0, 0, 0, 0, 0] ("Keys 2") u8[] [0, 1, 0, 0, 0, 0, 0, 0, 0, 0, 0, 0, 0, 0, 0, 0] ("Keys 2") u8[] [0, 0, 1, 0, 0, 0, 0, 0, 0, 0, 0, 0, 0, 0, 0, 0] ("Keys 2") u8[] [0, 0, 0, 1, 0, 0, 0, 0, 0, 0, 0, 0, 0, 0, 0, 0] ("Keys 2") u8[] [0, 0, 0, 0, 0, 0, 0, 0, 0, 0, 0, 0, 1, 0, 0, 0] ("Keys 2") u8[] [0, 0, 0, 0, 1, 0, 0, 0, 0, 0, 0, 0, 0, 0, 0, 0] ("Keys 2") u8[] [0, 0, 0, 0, 0, 1, 0, 0, 0, 0, 0, 0, 0, 0, 0, 0] ("Keys 2") u8[] [0, 0, 0, 0, 0, 0, 1, 0, 0, 0, 0, 0, 0, 0, 0, 0] ("Keys 2") u8[] [0, 0, 0, 0, 0, 0, 0, 0, 0, 0, 0, 0, 0, 1, 0, 0] ("Keys 2") u8[] [0, 0, 0, 0, 0, 0, 0, 1, 0, 0, 0, 0, 0, 0, 0, 0] ("Keys 2") u8[] [0, 0, 0, 0, 0, 0, 0, 0, 1, 0, 0, 0, 0, 0, 0, 0] ("Keys 2") u8[] [0, 0, 0, 0, 0, 0, 0, 0, 0, 1, 0, 0, 0, 0, 0, 0] ("Keys 2") u8[] [0, 0, 0, 0, 0, 0, 0, 0, 0, 0, 0, 0, 0, 0, 1, 0] ("Keys 2") u8[] [0, 0, 0, 0, 0, 0, 0, 0, 0, 0, 1, 0, 0, 0, 0, 0] ("Keys 2") u8[] [1, 0, 0, 0, 0, 0, 0, 0, 0, 0, 0, 0, 0, 0, 0, 0] ("Keys 2") u8[] [0, 0, 0, 0, 0, 0, 0, 0, 0, 0, 0, 1, 0, 0, 0, 0] ("Keys 2") u8[] [0, 0, 0, 0, 0, 0, 0, 0, 0, 0, 0, 0, 0, 0, 0, 1] ("Keys 2")] -> w619
                frame 0, Default {
                }
                frame 49 {
                  # "1 = 1"
                }
                frame 50 {
                  # "2 = 2"
                }
                frame 51 {
                  # "3 = 3"
                }
                frame 52 {
                  # "4 =C"
                }
                frame 113 {
                  # "Q = 4"
                }
                frame 119 {
                  # "W = 5"
                }
                frame 101 {
                  # "E = 6"
                }
                frame 114 {
                  # "R = D"
                }
                frame 97 {
                  # "A = 7"
                }
                frame 115 {
                  # "S = 8"
                }
                frame 100 {
                  # "D = 9"
                }
                frame 102 {
                  # "F = E"
                }
                frame 122 {
                  # "Z = A"
                }
                frame 120 {
                  # "X = 0"
                }
                frame 99 {
                  # "C = B"
                }
                frame 118 {
                  # "V = F"
                }
              }
            }
          }
          n331 = for {
            tunnel: [w638] -> w617
            tunnel: [w640] -> w616
            tunnel: w615 -> [w639] mode=indexing
            i -> [w640]
            stop <- w638 stop-if-true
            # "Key"
            n332 = Equal?(x=w639, y=u8 1) -> (x = y?=w638:bool)
          }
        }
        n333 = Unbundle By Name(w602) -> ("PC"=w607:u16, "V Registers"=w612:u8[], "Opcode"=w614:u16)
        n334 = Increment(x=w607) -> (x+1=w606:u16)
        n335 = call "Opcode at X.vi"("X Position"=enum16{"First", "Second", "Third", "Fourth"}."Second", "Opcode"=w614) -> ("Opcode at X Position (U8)"=w611:u8)  [unwired: 9 in]
        n336 = Increment(x=w606) -> (x+1=w605:u16)
        n337 = To Long Integer(number=w611) -> (32bit integer=w610:i32)
        n338 = To Unsigned Byte Integer(number=w601) -> (unsigned 8bit integer=w609:u8)
        n339 = Replace Array Subset(array=w612, new element=w609, index=w610) -> (w604:u8[])
        n340 = Bundle By Name(cluster=w602, "PC"=w605, "V Registers"=w604) -> (w608:T2)
      }
      frame "FX15: Set Delay Timer to VX" {
        # "// FX15 - Sets the delay timer to VX\n                case 0x0015:\n                    delay_timer = V[(opcode & 0x0F00) >> 8];\n                    pc += 2;\n                    break;"
        n341 = Unbundle By Name(w652) -> ("PC"=w650:u16, "V Registers"=w645:u8[], "Opcode"=w647:u16)
        n342 = Increment(x=w650) -> (x+1=w649:u16)
        n343 = call "Opcode at X.vi"("X Position"=enum16{"First", "Second", "Third", "Fourth"}."Second", "Opcode"=w647) -> ("Opcode at X Position (U8)"=w644:u8)  [unwired: 9 in]
        n344 = Increment(x=w649) -> (x+1=w648:u16)
        n345 = To Long Integer(number=w644) -> (32bit integer=w643:i32)
        n346 = Index Array(array=w645, index=w643) -> (element=w642:u8)
        n347 = Bundle By Name(cluster=w652, "PC"=w648, "DelayTimer"=w642) -> (w653:T2)
      }
      frame "FX18: Set SoundTimer to VX" {
        # "// FX18 - Sets the sound timer to VX\n                case 0x0018:\n                    sound_timer = V[(opcode & 0x0F00) >> 8];\n                    pc += 2;\n                    break;"
        n348 = Unbundle By Name(w657) -> ("PC"=w665:u16, "V Registers"=w661:u8[], "Opcode"=w663:u16)
        n349 = Increment(x=w665) -> (x+1=w664:u16)
        n350 = call "Opcode at X.vi"("X Position"=enum16{"First", "Second", "Third", "Fourth"}."Second", "Opcode"=w663) -> ("Opcode at X Position (U8)"=w660:u8)  [unwired: 9 in]
        n351 = Increment(x=w664) -> (x+1=w656:u16)
        n352 = To Long Integer(number=w660) -> (32bit integer=w659:i32)
        n353 = Index Array(array=w661, index=w659) -> (element=w655:u8)
        n354 = Bundle By Name(cluster=w657, "PC"=w656, "SoundTimer"=w655) -> (w658:T2)
      }
      frame "FX1E: Add VX to I" {
        # "// FX1E - Adds VX to I\n                case 0x001E:\n                    // VF is set to 1 when range overflow (I+VX>0xFFF), and 0\n                    // when there isn't.\n                    if(I + V[(opcode & 0x0F00) >> 8] > 0xFFF)\n                        V[0xF] = 1;\n                    else\n                        V[0xF] = 0;\n                    I += V[(opcode & 0x0F00) >> 8];\n                    pc += 2;\n                    break;"
        n355 = Unbundle By Name(w685) -> ("PC"=w687:u16, "V Registers"=w675:u8[], "Opcode"=w678:u16, "I"=w682:u16)
        n356 = Increment(x=w687) -> (x+1=w688:u16)
        n357 = call "Opcode at X.vi"("X Position"=enum16{"First", "Second", "Third", "Fourth"}."Second", "Opcode"=w678) -> ("Opcode at X Position (U8)"=w679:u8)  [unwired: 9 in]
        n358 = Increment(x=w688) -> (x+1=w684:u16)
        n359 = To Long Integer(number=w679) -> (32bit integer=w677:i32)
        n360 = Index Array(array=w675, index=w677) -> (element=w683:u8)
        n361 = To Unsigned Word Integer(number=w683) -> (unsigned 16bit integer=w676:u16)
        n362 = Add(x=w676, y=w682) -> (x+y=w672:u16)
        n363 = Greater?(x=w672, y=u16 4095) -> (0:w671:bool)
        n364 = Select(t=u8 1, s=w671, f=u8 0) -> (s? t:f=w670:u8)
        n365 = To Long Integer(number=u8 15) -> (32bit integer=w673:i32)
        n366 = Replace Array Subset(array=w675, new element=w670, index=w673) -> (w667:u8[])
        n367 = Bundle By Name(cluster=w685, "PC"=w684, "I"=w672, "V Registers"=w667) -> (w686:T2)
      }
      frame "FX29: Set Loc of Sprite for VX" {
        # "// FX29 - Sets I to the location of the sprite for the\n                // character in VX. Characters 0-F (in hexadecimal) are\n                // represented by a 4x5 font\n                case 0x0029:\n                    I = V[(opcode & 0x0F00) >> 8] * 0x5;\n                    pc += 2;\n                    break;"
        # "#Doublecheck the math and conversions here"
        n368 = Unbundle By Name(w702) -> ("PC"=w701:u16, "V Registers"=w695:u8[], "Opcode"=w697:u16)
        n369 = Increment(x=w701) -> (x+1=w700:u16)
        n370 = call "Opcode at X.vi"("X Position"=enum16{"First", "Second", "Third", "Fourth"}."Second", "Opcode"=w697) -> ("Opcode at X Position (U8)"=w694:u8)  [unwired: 9 in]
        n371 = Increment(x=w700) -> (x+1=w699:u16)
        n372 = To Long Integer(number=w694) -> (32bit integer=w693:i32)
        n373 = Index Array(array=w695, index=w693) -> (element=w690:u8)
        n374 = Multiply(x=w690, y=u8 5) -> (x*y=w692:u8)
        n375 = To Unsigned Word Integer(number=w692) -> (unsigned 16bit integer=w691:u16)
        n376 = Bundle By Name(cluster=w702, "PC"=w699, "I"=w691) -> (w703:T2)
      }
      frame "FX33: Store BCD of VX" {
        # "// FX33 - Stores the Binary-coded decimal representation of VX\n                // at the addresses I, I plus 1, and I plus 2\n                case 0x0033:\n                    memory[I]     = V[(opcode & 0x0F00) >> 8] / 100;\n                    memory[I + 1] = (V[(opcode & 0x0F00) >> 8] / 10) % 10;\n                    memory[I + 2] = (V[(opcode & 0x0F00) >> 8] % 100) % 10;\n                    pc += 2;\n                    break;"
        # "middle sig digit"
        # "Stores the binary-coded decimal representation of VX, with the most significant of three digits at the address in I, the middle digit at I plus 1, and\n the least significant digit at I plus 2. (In other words, take the decimal representation of VX, place the hundreds digit in memory at location in I, \nthe tens digit at location I+1, and the ones digit at location I+2.)"
        # "least significant digit"
        # "most significant digit"
        n377 = Unbundle By Name(w735) -> ("PC"=w734:u16, "Memory"=w712:u8[], "I"=w711:u16, "V Registers"=w728:u8[], "Opcode"=w730:u16)
        n378 = Increment(x=w734) -> (x+1=w733:u16)
        n379 = call "Opcode at X.vi"("X Position"=enum16{"First", "Second", "Third", "Fourth"}."Second", "Opcode"=w730) -> ("Opcode at X Position (U8)"=w727:u8)  [unwired: 9 in]
        n380 = Increment(x=w733) -> (x+1=w732:u16)
        n381 = To Long Integer(number=w727) -> (32bit integer=w726:i32)
        n382 = Index Array(array=w728, index=w726) -> (element=w704:u8)
        n383 = To Long Integer(number=w711) -> (32bit integer=w710:i32)
        n384 = To Double Precision Float(number=w704) -> (double precision float=w718:dbl)
        n385 = Divide(x=w718, y=10.0) -> (x/y=w722:dbl)
        n386 = Quotient & Remainder(x=w718, y=100.0) -> (floor(x/y)=w724:dbl)  [unwired: 1 out]
        n387 = Quotient & Remainder(x=w718, y=100.0) -> (x-y*floor(x/y)=w714:dbl)  [unwired: 1 out]
        n388 = To Unsigned Byte Integer(number=w724) -> (unsigned 8bit integer=w709:u8)
        n389 = Quotient & Remainder(x=w722, y=10.0) -> (x-y*floor(x/y)=w720:dbl)  [unwired: 1 out]
        n390 = Quotient & Remainder(x=w714, y=10.0) -> (x-y*floor(x/y)=w713:dbl)  [unwired: 1 out]
        n391 = Round Toward -Infinity(1:w720) -> (0:w719:dbl)
        n392 = Round Toward -Infinity(1:w713) -> (0:w715:dbl)
        n393 = To Unsigned Byte Integer(number=w719) -> (unsigned 8bit integer=w708:u8)
        n394 = To Unsigned Byte Integer(number=w715) -> (unsigned 8bit integer=w707:u8)
        n395 = Build Array(w709, w708, w707) -> (w706:u8[])
        n396 = Replace Array Subset(array=w712, new element=w706, index=w710) -> (w705:u8[])
        n397 = Bundle By Name(cluster=w735, "PC"=w732, "Memory"=w705) -> (w736:T2)
      }
      frame "FX55: Store V0 to VX" {
        # "// FX55 - Stores V0 to VX in memory starting at address I\n                case 0x0055:\n                    for (int i = 0; i <= ((opcode & 0x0F00) >> 8); ++i)\n                        memory[I + i] = V[i];\n\n                    // On the original interpreter, when the\n                    // operation is done, I = I + X + 1.\n                    I += ((opcode & 0x0F00) >> 8) + 1;\n                    pc += 2;\n                    break;"
        # "#doublecheck conversions"
        n398 = Unbundle By Name(w754) -> ("PC"=w752:u16, "Memory"=w747:u8[], "I"=w741:u16, "V Registers"=w744:u8[], "Opcode"=w748:u16)
        n399 = call "Opcode at X.vi"("X Position"=enum16{"First", "Second", "Third", "Fourth"}."Second", "Opcode"=w748) -> ("Opcode at X Position (U8)"=w740:u8)  [unwired: 9 in]
        n400 = To Long Integer(number=w740) -> (32bit integer=w745:i32)
        n401 = To Unsigned Word Integer(number=w740) -> (unsigned 16bit integer=w739:u16)
        n402 = Increment(x=w752) -> (x+1=w751:u16)
        n403 = Add(x=w741, y=w739) -> (x+y=w738:u16)
        n404 = for {
          N: w745 -> [_]
          tunnel: w744 -> [w758]
          tunnel: [w757] -> w743 mode=indexing
          i -> [w756]
          n405 = Index Array(array=w758, index=w756) -> (element=w757:u8)
        }
        n406 = Increment(x=w751) -> (x+1=w750:u16)
        n407 = To Long Integer(number=w741) -> (32bit integer=w746:i32)
        n408 = Increment(x=w738) -> (x+1=w737:u16)
        n409 = Replace Array Subset(array=w747, new element=w743, index=w746) -> (w742:u8[])
        n410 = Bundle By Name(cluster=w754, "PC"=w750, "Memory"=w742, "I"=w737) -> (w755:T2)
      }
      frame "FX65: Fill V0 to VX" {
        # "case 0x0065:\n                    for (int i = 0; i <= ((opcode & 0x0F00) >> 8); ++i)\n                        V[i] = memory[I + i];\n\n                    // On the original interpreter,\n                    // when the operation is done, I = I + X + 1.\n                    I += ((opcode & 0x0F00) >> 8) + 1;\n                    pc += 2;\n                    break;"
        n411 = Unbundle By Name(w771) -> ("PC"=w767:u16, "Opcode"=w777:u16, "V Registers"=w774:u8[], "I"=w763:u16, "Memory"=w775:u8[])
        n412 = Increment(x=w767) -> (x+1=w768:u16)
        n413 = call "Opcode at X.vi"("X Position"=enum16{"First", "Second", "Third", "Fourth"}."Second", "Opcode"=w777) -> ("Opcode at X Position (U8)"=w762:u8)  [unwired: 9 in]
        n414 = Increment(x=w768) -> (x+1=w766:u16)
        n415 = To Long Integer(number=w763) -> (32bit integer=w765:i32)
        n416 = To Long Integer(number=w762) -> (32bit integer=w764:i32)
        n417 = To Unsigned Word Integer(number=w762) -> (unsigned 16bit integer=w761:u16)
        n418 = Add(x=w763, y=w761) -> (x+y=w760:u16)
        n419 = Array Subset(array=w775, index=w765, length=w764) -> (w772:u8[])
        n420 = Increment(x=w760) -> (x+1=w759:u16)
        n421 = Replace Array Subset(array=w774, new element=w772, index=0) -> (w769:u8[])
        n422 = Bundle By Name(cluster=w771, "PC"=w766, "V Registers"=w769, "I"=w759) -> (w770:T2)
      }
      frame "Debug: Opcode Not Done Yet" {
        n423 = Unbundle By Name(w783) -> ("Opcode"=w782:u16)
        n424 = Format Into String(format string="%04x", initial string="Opcode: ", w782) -> (resulting string=w781:string)  [unwired: 1 in, 1 out]
        n425 = One Button Dialog(message=w781, button name ("OK")="Not Yet Implemented" ("message")) -> ()  [unwired: 1 out]
      }
    }
    n426 = Unbundle By Name(w10) -> ("SoundTimer"=w14:u8, "DelayTimer"=w11:u8)  [unwired: 4 out]
    n427 = call "Timing Engine.vi"() -> ()  [unwired: 9 in, 3 out]
    n428 = Decrement(x=w14) -> (x-1=w15:u8)
    n429 = Decrement(x=w11) -> (x-1=w12:u8)
    n430 = Greater Than 0?(x=w11) -> (x > 0?=w13:bool)
    n431 = Greater Than 0?(x=w14) -> (x > 0?=w16:bool)
    n432 = Select(t=w15, s=w16, f=w14) -> (s? t:f=w8:u8)
    n433 = Select(t=w12, s=w13, f=w11) -> (s? t:f=w7:u8)
    n434 = Bundle By Name(cluster=w10, "SoundTimer"=w8, "DelayTimer"=w7) -> (w9:T2)
  }
